vi "DBM Reg proc_temp.vi"(4 "Calfunc ?":bool, 6 "배열":u32[](array[numeric]), 7 "Query info":T1, 8 "에러 입력":errorcluster caption="에러 입력(에러 없음)", 9 "CMC":string[][](array[string]), 10 "calfunc":string[][](array[string]), 11 "Proc 참조 in":refnum<vi>) -> (0 "에러 출력":errorcluster, 2 "배열출력":string[][](array[string]), 3 "에러?":bool)   [LabVIEW 2020]
uses:
  Controls/Clst_Query Info.ctl
  Public/Polymorph/Array Dedup_2D Str.vi
  Public/Polymorph/Array Dedup_1D Str.vi
  <vilib>/Utility/error.llb/Error Cluster From Error Code.vi
  Public/Polymorph/Cell Space_Table.vi
  <vilib>/ErrorRing/Error Ring.xnode
panel:
  out "값":string[][](array[string])
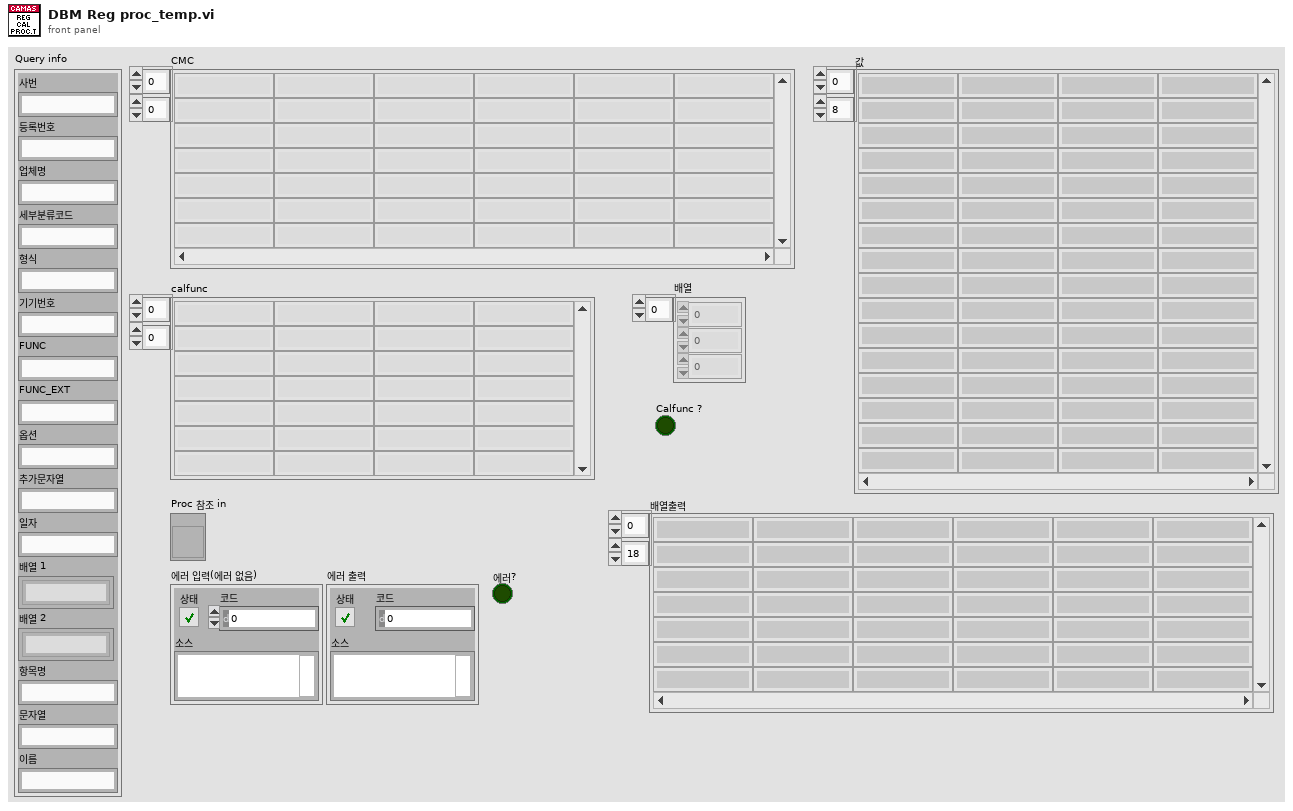
[diagram p1: front panel]
types:
  T1 = typedef "Clst_Query Info.ctl" = cluster{"사번":string, "등록번호":string, "업체명":string, "세부분류코드":string, "형식":string, "기기번호":string, "FUNC":string, "FUNC_EXT":string, "옵션":string, "추가문자열":string, "일자":string, "배열 1":string[], "배열 2":string[], "항목명":string, "문자열":string, "이름":string}
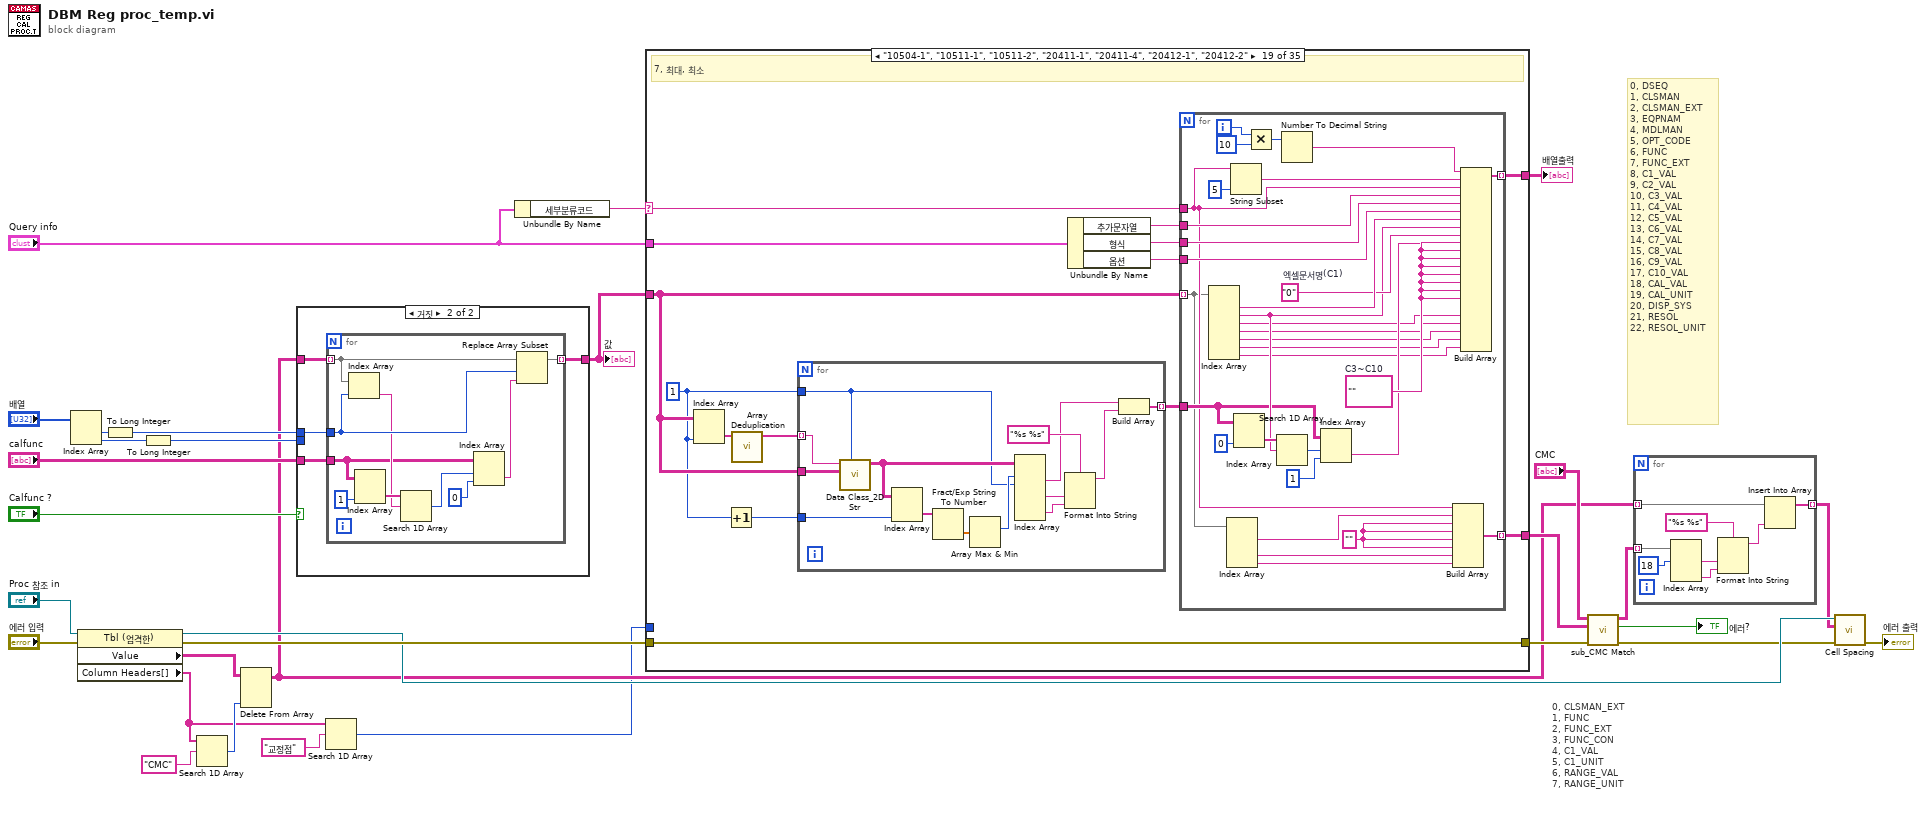
[diagram p0: block diagram]
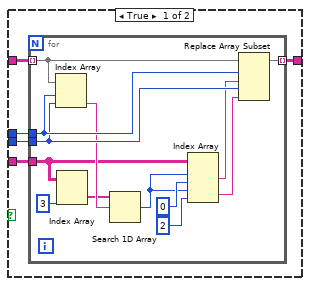
[diagram p2: hidden frame]
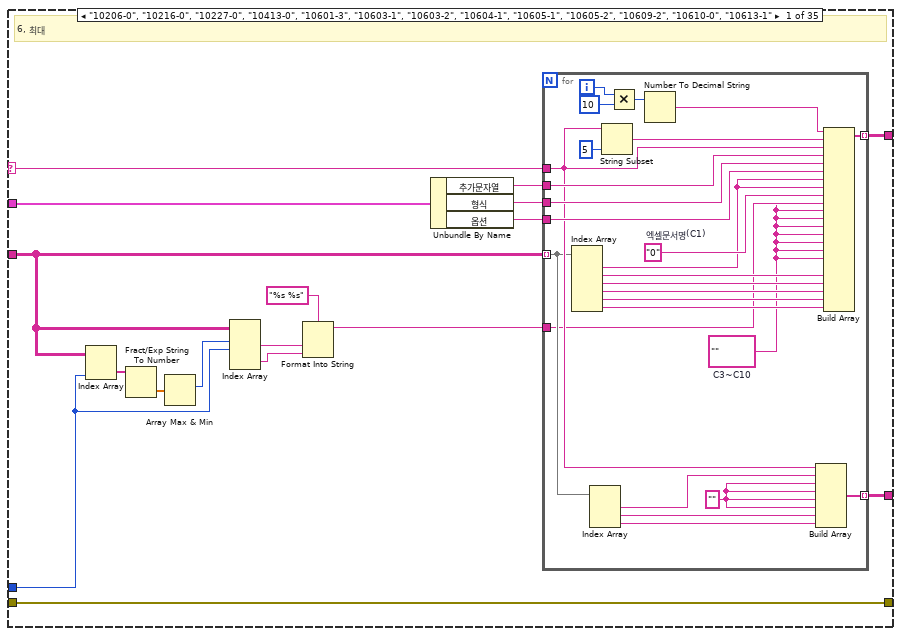
[diagram p3: hidden frame]
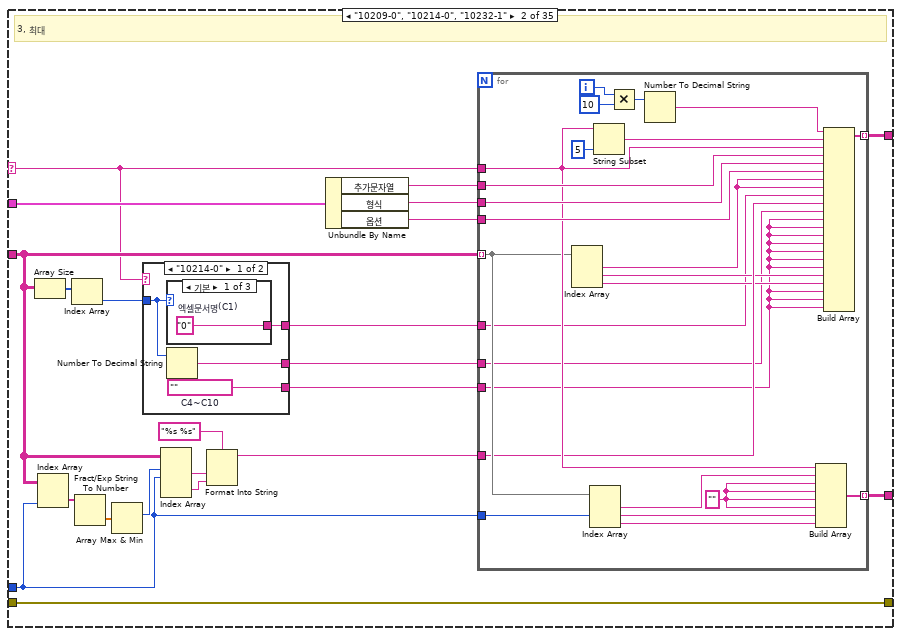
[diagram p4: hidden frame]
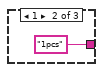
[diagram p5: hidden frame]
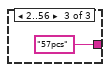
[diagram p6: hidden frame]
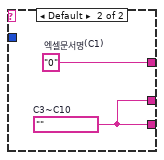
[diagram p7: hidden frame]
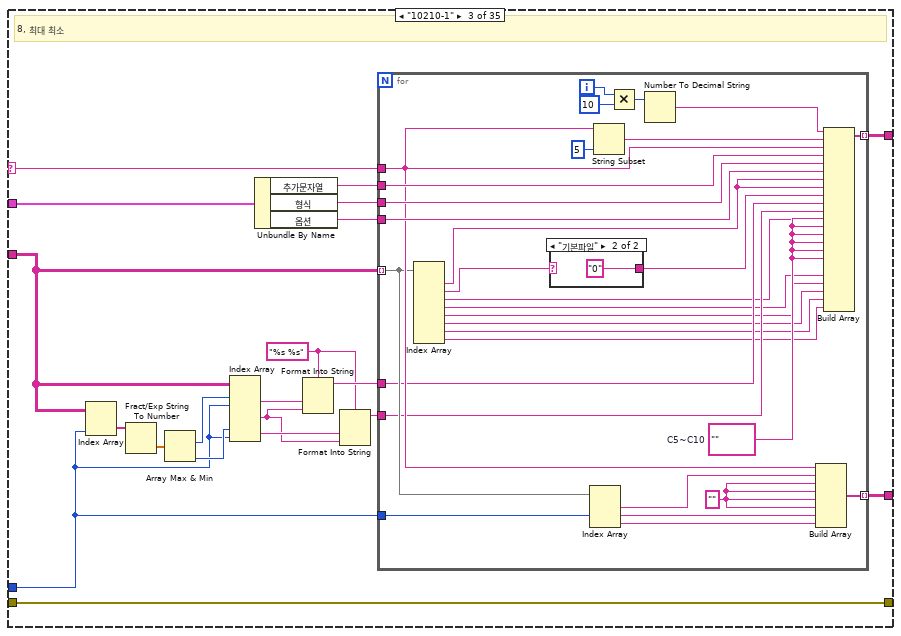
[diagram p8: hidden frame]
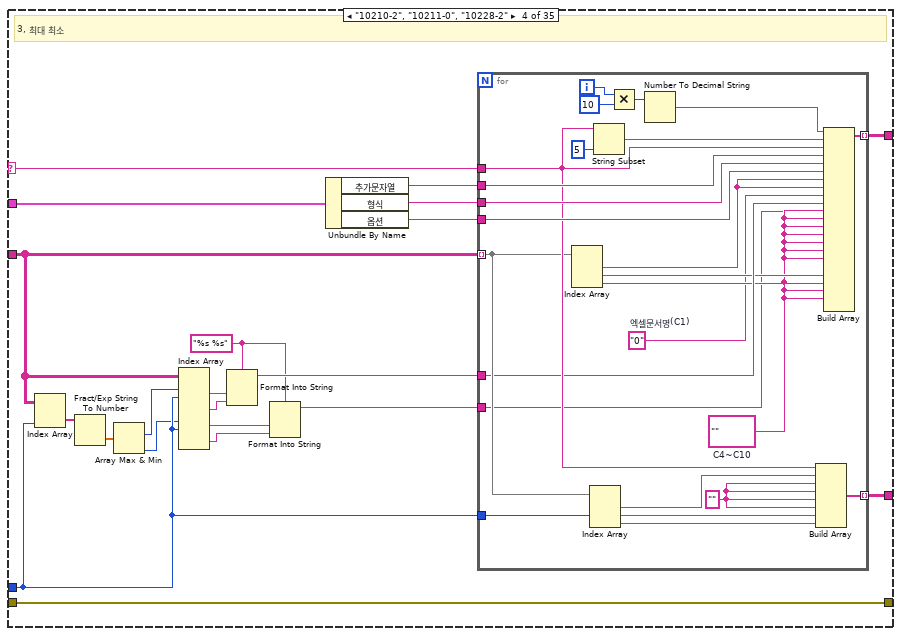
[diagram p10: hidden frame]
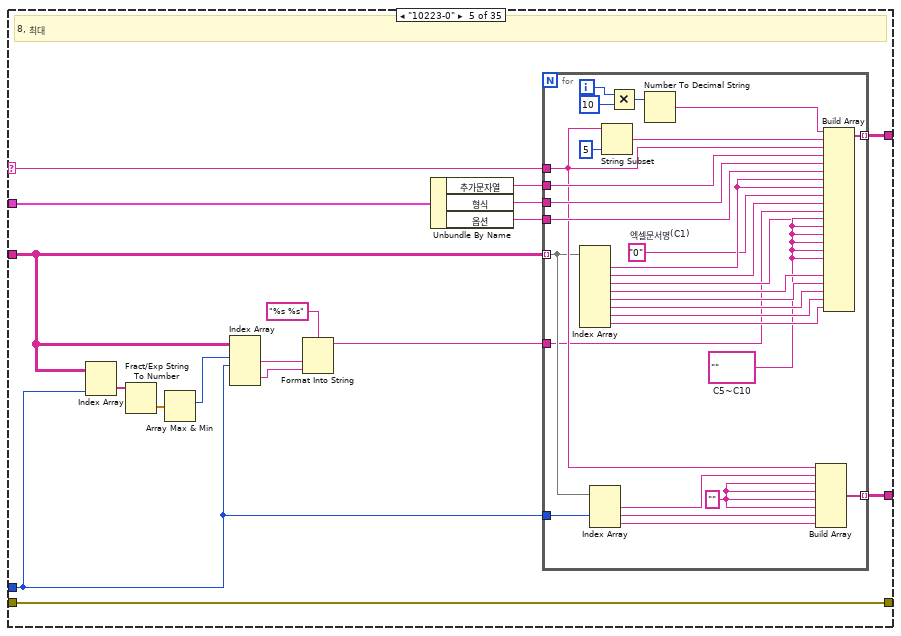
[diagram p11: hidden frame]
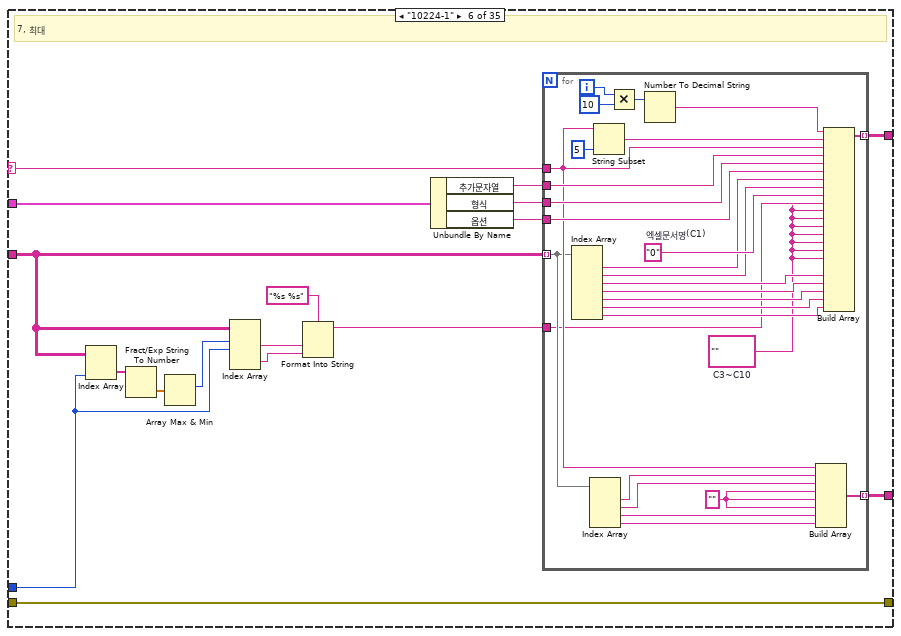
[diagram p12: hidden frame]
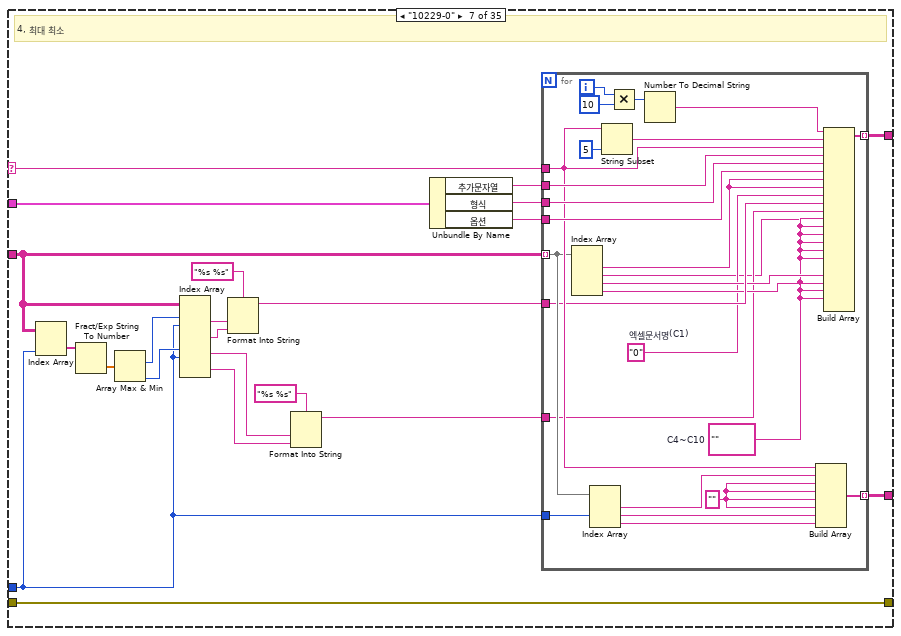
[diagram p13: hidden frame]
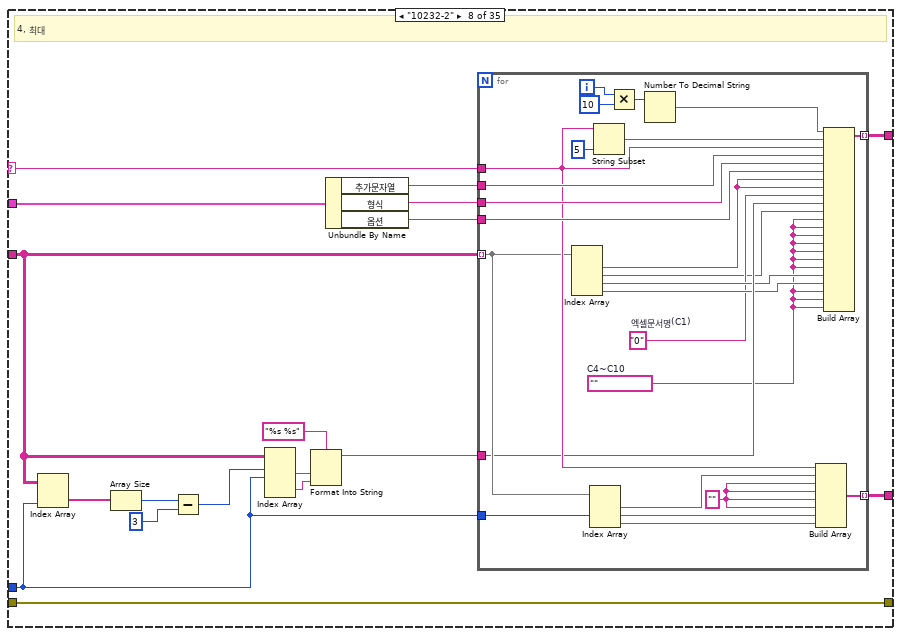
[diagram p14: hidden frame]
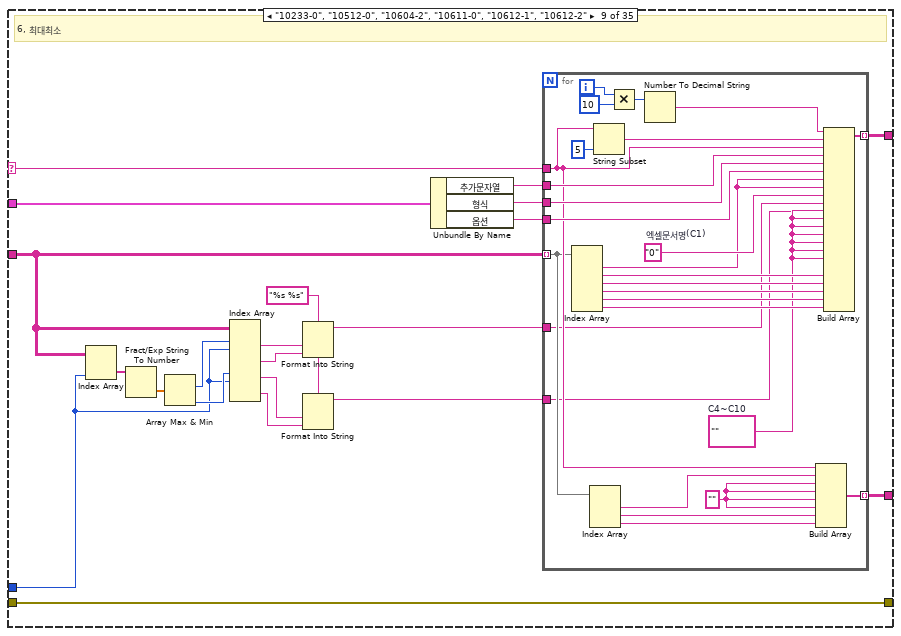
[diagram p15: hidden frame]
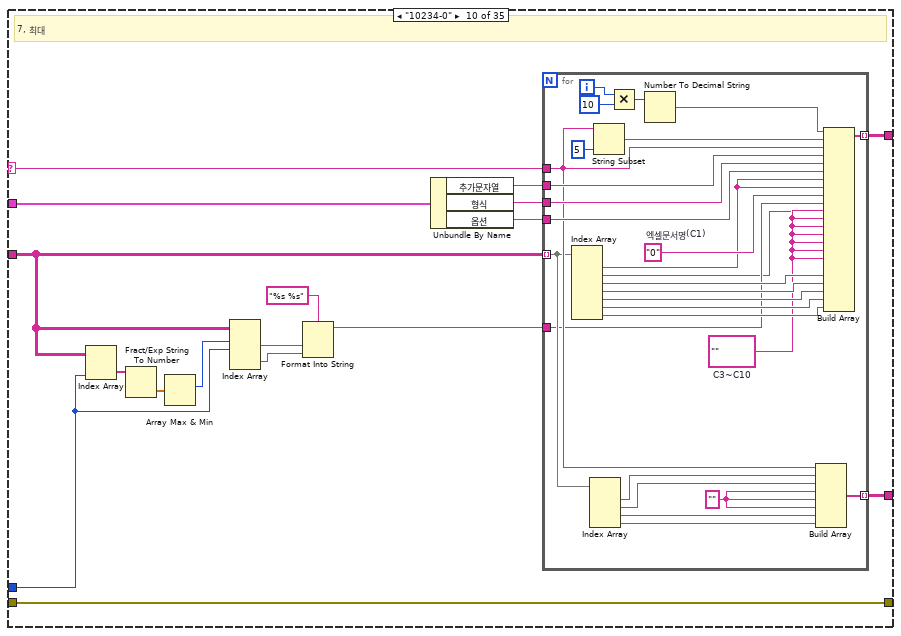
[diagram p16: hidden frame]
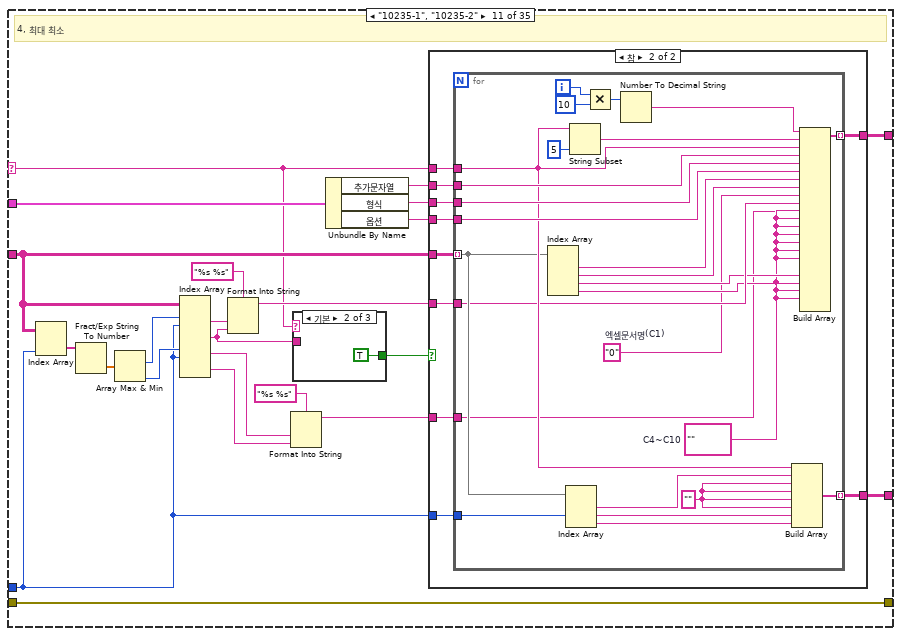
[diagram p17: hidden frame]
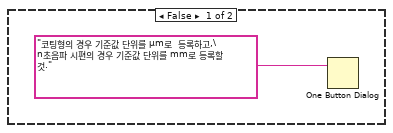
[diagram p18: hidden frame]
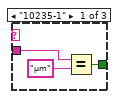
[diagram p19: hidden frame]
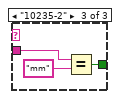
[diagram p20: hidden frame]
diagram:
  # "0, CLSMAN_EXT\n1, FUNC\n2, FUNC_EXT\n3, FUNC_CON\n4, C1_VAL\n5, C1_UNIT\n6, RANGE_VAL\n7, RANGE_UNIT"
  # "0, DSEQ\n1, CLSMAN\n2, CLSMAN_EXT\n3, EQPNAM\n4, MDLMAN\n5, OPT_CODE\n6, FUNC\n7, FUNC_EXT\n8, C1_VAL\n9, C2_VAL\n10, C3_VAL\n11, C4_VAL\n12, C5_VAL\n13, C6_VAL\n14, C7_VAL\n15, C8_VAL\n16, C9_VAL\n17, C10_VAL\n18, CAL_VAL\n19, CAL_UNIT\n20, DISP_SYS\n21, RESOL\n22, RESOL_UNIT"
  n1 = Index Array(array="배열") -> (element #1=w12:u32, element #2=w11:u32)  [unwired: 2 in]
  n2 = property class="Tbl (엄격한)"(reference="Proc 참조 in", error in="에러 입력") -> (reference out=w24:refnum<vi>, error out=w27:errorcluster, "Value"=w4:string[][], "Column Headers[]"=w2:string[])
  n3 = To Long Integer(number=w12) -> (32bit integer=w9:i32)
  n4 = To Long Integer(number=w11) -> (32bit integer=w8:i32)
  n5 = Search 1D Array(1D array=w2, element="CMC" ("원소")) -> (index of element=w22:i32)  [unwired: 1 in]
  n6 = Delete From Array(array=w4, index (col)=w22) -> (array with subset deleted=w5:string[][])  [unwired: 2 in, 1 out]
  n7 = case shown="거짓" "Calfunc ?" {
    tunnel: "calfunc" -> [w35 w52]
    tunnel: w5 -> [w34 w51]
    tunnel: w9 -> [w33 w50]
    tunnel: w8 -> [w32 _]
    tunnel: [w31 w49] -> w6
    frame True {
      n8 = for {
        tunnel: w34 -> [w43] mode=indexing
        tunnel: w35 -> [w42]
        tunnel: [w48] -> w31 mode=indexing
        tunnel: w33 -> [w47]
        tunnel: w32 -> [w46]
        n9 = Index Array(array=w43, index #1=w47, index #2=w46) -> (element #2=w45:string)  [unwired: 1 out]
        n10 = Index Array(array=w42, index (col)=3 ("인덱스 (열)")) -> (element=w44:string[])  [unwired: 1 in]
        n11 = Search 1D Array(1D array=w44, element=w45) -> (index of element=w36:i32)  [unwired: 1 in]
        n12 = Index Array(array=w42, index (row) #1=w36, index (col) #1=0 ("비활성화된 인덱스 (열)"), index (row) #2=w36, index (col) #2=2 ("비활성화된 인덱스 (열)")) -> (element #1=w40:string, element #2=w39:string)
        n13 = Replace Array Subset(array=w43, new element #1=w40, index #1=w47, new element #2=w39, index #2=w46) -> (w48:string[])
      }
    }
    frame False {
      n14 = for {
        tunnel: w51 -> [w58] mode=indexing
        tunnel: w52 -> [w57]
        tunnel: [w62] -> w49 mode=indexing
        tunnel: w50 -> [w61]
        n15 = Index Array(array=w58, index=w61) -> (element=w59:string)
        n16 = Index Array(array=w57, index (col)=1 ("비활성화된 인덱스 (열)")) -> (element=w60:string[])  [unwired: 1 in]
        n17 = Search 1D Array(1D array=w60, element=w59) -> (index of element=w56:i32)  [unwired: 1 in]
        n18 = Index Array(array=w57, index (row)=w56, index (col)=0 ("비활성화된 인덱스 (열)")) -> (element=w54:string)
        n19 = Replace Array Subset(array=w58, new element=w54, index=w61) -> (w62:string[])
      }
    }
  }
  "값" <- w6
  n20 = Search 1D Array(1D array=w2, element="교정점" ("원소")) -> (index of element=w1:i32)  [unwired: 1 in]
  n21 = Unbundle By Name("Query info") -> ("세부분류코드"=w28:string)
  n22 = case shown="\"10504-1\", \"10511-1\", \"10511-2\", \"20411-1\", \"20411-4\", \"20412-1\", \"20412-2\"" w28 {
    selector: w28 -> [w74 w109 w176 w229 w271 w317 w356 w403 w457 w501 w541 w613 w659 w706 w760 w849 w886 w927 w991 w1055 w1119 w1157 w1216 w1250 w1308 w1413 w1481 w1546 w1611 w1683 w1755 w1822 w1882 w1942 w1979]
    tunnel: [w72 w121 w174 w227 w269 w315 w366 w410 w455 w499 w551 w611 w657 w704 w758 w847 w884 w926 w989 w1053 w1117 w1155 w1214 w1248 w1306 w1411 w1479 w1544 w1609 w1681 w1753 w1820 w1880 w1940 w1981] -> w20
    tunnel: w27 -> [w72 w121 w174 w227 w269 w315 w366 w410 w455 w499 w551 w611 w657 w704 w758 w847 w884 w926 w989 w1053 w1117 w1155 w1214 w1248 w1306 w1411 w1479 w1544 w1609 w1681 w1753 w1820 w1880 w1940 _]
    tunnel: "Query info" -> [w79 w127 w181 w234 w276 w322 w372 w416 w462 w506 w557 w618 w664 w711 w765 w854 w891 w929 w1000 w1060 w1124 w1166 w1222 w1256 w1316 w1422 w1490 w1555 w1620 w1692 w1764 w1831 w1891 w1948 _]
    tunnel: w6 -> [w69 w112 w171 w225 w265 w311 w358 w404 w452 w495 w543 w607 w653 w700 w743 w846 w883 w923 w995 w1050 w1109 w1161 w1218 w1252 w1297 w1417 w1485 w1550 w1615 w1687 w1759 w1826 w1886 w1944 _]
    tunnel: [w75 w123 w177 w230 w272 w318 w368 w412 w458 w502 w553 w614 w660 w707 w761 w850 w887 w928 w992 w1056 w1120 w1158 w1217 w1251 w1309 w1414 w1482 w1547 w1612 w1684 w1756 w1823 w1883 w1943 _] -> w30
    tunnel: [w73 w122 w175 w228 w270 w316 w367 w411 w456 w500 w552 w612 w658 w705 w759 w848 w885 w915 w990 w1054 w1118 w1156 w1215 w1249 w1307 w1412 w1480 w1545 w1610 w1682 w1754 w1821 w1881 w1941 string[][] [] ("Value")] -> w16
    tunnel: w1 -> [w63 w114 w162 w219 w260 w306 w353 w405 w442 w490 w537 w602 w648 w695 w751 _ _ w925 _ w1051 w1108 _ _ _ _ _ _ _ _ _ _ _ _ _ _]
    frame "10206-0", "10216-0", "10227-0", "10413-0", "10601-3", "10603-1", "10603-2", "10604-1", "10605-1", "10605-2", "10609-2", "10610-0", "10613-1" {
      # "6, 최대"
      n23 = Index Array(array=w69, index (col)=w63) -> (element=w70:string[])  [unwired: 1 in]
      n24 = Fract/Exp String To Number(string=w70) -> (number=w71:dbl[])  [unwired: 3 in, 1 out]
      n25 = Array Max & Min(array=w71) -> (max index (indices)=w68:i32)  [unwired: 3 out]
      n26 = Index Array(array=w69, index (row) #1=w68, index (col) #1=w63) -> (element #1=w67:string, element #2=w64:string)  [unwired: 2 in]
      n27 = Format Into String(format string="%s %s" ("포맷 문자열"), w67, w64) -> (resulting string=w66:string)  [unwired: 2 in, 1 out]
      n28 = Unbundle By Name(w79) -> ("추가문자열"=w78:string, "형식"=w77:string, "옵션"=w76:string)
      n29 = for {
        tunnel: w69 -> [w88] mode=indexing
        tunnel: w74 -> [w89]
        tunnel: w78 -> [w98]
        tunnel: w77 -> [w97]
        tunnel: w76 -> [w96]
        tunnel: [w87] -> w73 mode=indexing
        tunnel: w66 -> [w84]
        tunnel: [w99] -> w75 mode=indexing
        i -> [w105]
        w85 = "" ("원소")
        w80 = ""  # C3~C10
        w95 = "0"  # 엑셀문서명(C1)
        n30 = Index Array(array=w88) -> (element #1=w83:string, element #2=w94:string, element #3=w93:string, element #4=w92:string, element #5=w91:string, element #6=w90:string)  [unwired: 6 in]
        n31 = Index Array(array=w88) -> (element #1=w86:string, element #2=w82:string, element #3=w81:string)  [unwired: 3 in]
        n32 = String Subset(string=w89, length (rest)=5 ("길이(나머지)")) -> (substring=w100:string)  [unwired: 1 in]
        n33 = Multiply(x=w105, y=10) -> (x*y=w103:i32)
        n34 = Number To Decimal String(number=w103) -> (decimal integer string=w102:string)  [unwired: 1 in]
        n35 = Build Array(w89, w86, w85, w85, w85, w85, w82, w81) -> (w87:string[])
        n36 = Build Array(w102, w100, w89, w98, w97, w96, w83, w83, w95, w84, w80, w80, w80, w80, w80, w80, w80, w80, w94, w93, w92, w91, w90) -> (w99:string[])
      }
    }
    frame "10209-0", "10214-0", "10232-1" {
      # "3, 최대"
      n37 = Array Size(array=w112) -> (size(s)=w111:i32[])
      n38 = Index Array(array=w112, index (col)=w114) -> (element=w113:string[])  [unwired: 1 in]
      n39 = Index Array(array=w111) -> (element=w110:i32)  [unwired: 1 in]
      n40 = Fract/Exp String To Number(string=w113) -> (number=w120:dbl[])  [unwired: 3 in, 1 out]
      n41 = Array Max & Min(array=w120) -> (max index (indices)=w118:i32)  [unwired: 3 out]
      n42 = case shown="\"10214-0\"" w109 {
        tunnel: [w131 w135] -> w108
        tunnel: [w130 w135] -> w106
        tunnel: w110 -> [w129 _]
        tunnel: [w128 w136] -> w107
        frame "10214-0" {
          w130 = ""  # C4~C10
          n43 = case shown="기본" w129 {
            tunnel: [w132 "1pcs" ("엑셀문서명(C1)") "57pcs" ("엑셀문서명(C1)")] -> w128
            frame Default {
              w132 = "0"  # 엑셀문서명(C1)
            }
            frame 1 {
            }
            frame 2..56 {
            }
          }
          n44 = Number To Decimal String(number=w129) -> (decimal integer string=w131:string)  [unwired: 1 in]
        }
        frame Default {
          w136 = "0"  # 엑셀문서명(C1)
          w135 = ""  # C3~C10
        }
      }
      n45 = Index Array(array=w112, index (row) #1=w118, index (col) #1=w114) -> (element #1=w117:string, element #2=w116:string)  [unwired: 2 in]
      n46 = Format Into String(format string="%s %s" ("포맷 문자열"), w117, w116) -> (resulting string=w115:string)  [unwired: 2 in, 1 out]
      n47 = Unbundle By Name(w127) -> ("추가문자열"=w126:string, "형식"=w125:string, "옵션"=w124:string)
      n48 = for {
        tunnel: w112 -> [w150] mode=indexing
        tunnel: w109 -> [w151]
        tunnel: w126 -> [w154]
        tunnel: w125 -> [w153]
        tunnel: w124 -> [w152]
        tunnel: [w149] -> w122 mode=indexing
        tunnel: w115 -> [w147]
        tunnel: [w155] -> w123 mode=indexing
        tunnel: w114 -> [w144]
        tunnel: w108 -> [w139]
        tunnel: w107 -> [w138]
        tunnel: w106 -> [w137]
        i -> [w161]
        w143 = "" ("원소")
        n49 = Index Array(array=w150) -> (element #1=w142:string, element #2=w141:string, element #3=w140:string)  [unwired: 3 in]
        n50 = Index Array(array=w150, index #2=w144) -> (element #1=w148:string, element #2=w146:string, element #3=w145:string)  [unwired: 2 in]
        n51 = String Subset(string=w151, length (rest)=5 ("길이(나머지)")) -> (substring=w156:string)  [unwired: 1 in]
        n52 = Multiply(x=w161, y=10) -> (x*y=w159:i32)
        n53 = Number To Decimal String(number=w159) -> (decimal integer string=w158:string)  [unwired: 1 in]
        n54 = Build Array(w151, w148, w143, w143, w143, w143, w146, w145) -> (w149:string[])
        n55 = Build Array(w158, w156, w151, w154, w153, w152, w142, w142, w138, w147, w139, w137, w137, w137, w137, w137, w137, w137, w141, w140, w137, w137, w137) -> (w155:string[])
      }
    }
    frame "10210-1" {
      w166 = "%s %s" ("포맷 문자열")
      # "8, 최대 최소"
      n56 = Index Array(array=w171, index (col)=w162) -> (element=w172:string[])  [unwired: 1 in]
      n57 = Fract/Exp String To Number(string=w172) -> (number=w173:dbl[])  [unwired: 3 in, 1 out]
      n58 = Array Max & Min(array=w173) -> (max index (indices)=w170:i32, min index (indices)=w167:i32)  [unwired: 2 out]
      n59 = Index Array(array=w171, index (row) #1=w170, index (col) #1=w162, index (row) #3=w167, index (col) #3=w162) -> (element #1=w169:string, element #2=w164:string, element #3=w165:string)  [unwired: 2 in]
      n60 = Unbundle By Name(w181) -> ("추가문자열"=w180:string, "형식"=w179:string, "옵션"=w178:string)
      n61 = Format Into String(format string=w166, w169, w164) -> (resulting string=w168:string)  [unwired: 2 in, 1 out]
      n62 = Format Into String(format string=w166, w165, w164) -> (resulting string=w163:string)  [unwired: 2 in, 1 out]
      n63 = for {
        tunnel: w171 -> [w200] mode=indexing
        tunnel: w176 -> [w201]
        tunnel: w180 -> [w204]
        tunnel: w179 -> [w203]
        tunnel: w178 -> [w202]
        tunnel: [w199] -> w175 mode=indexing
        tunnel: w168 -> [w196]
        tunnel: [w205] -> w177 mode=indexing
        tunnel: w163 -> [w192]
        tunnel: w162 -> [w185]
        i -> [w211]
        w197 = "" ("원소")
        w195 = ""  # C5~C10
        n64 = Index Array(array=w200) -> (element #1=w184:string, element #2=w183:string, element #3=w191:string, element #4=w190:string, element #5=w189:string, element #6=w188:string, element #7=w187:string, element #8=w186:string)  [unwired: 8 in]
        n65 = case shown="\"기본파일\"" w183 {
          selector: w183 -> [w212 _]
          tunnel: [w212 "0" ("원소")] -> w182
          frame Default {
          }
          frame "기본파일" {
          }
        }
        n66 = Index Array(array=w200, index #2=w185) -> (element #1=w198:string, element #2=w194:string, element #3=w193:string)  [unwired: 2 in]
        n67 = String Subset(string=w201, length (rest)=5 ("길이(나머지)")) -> (substring=w206:string)  [unwired: 1 in]
        n68 = Multiply(x=w211, y=10) -> (x*y=w209:i32)
        n69 = Number To Decimal String(number=w209) -> (decimal integer string=w208:string)  [unwired: 1 in]
        n70 = Build Array(w201, w198, w197, w197, w197, w197, w194, w193) -> (w199:string[])
        n71 = Build Array(w208, w206, w201, w204, w203, w202, w184, w184, w182, w196, w192, w191, w195, w195, w195, w195, w195, w195, w190, w189, w188, w187, w186) -> (w205:string[])
      }
    }
    frame "10210-2", "10211-0", "10228-2" {
      w215 = "%s %s" ("포맷 문자열")
      # "3, 최대 최소"
      n72 = Index Array(array=w225, index (col)=w219) -> (element=w220:string[])  [unwired: 1 in]
      n73 = Fract/Exp String To Number(string=w220) -> (number=w226:dbl[])  [unwired: 3 in, 1 out]
      n74 = Array Max & Min(array=w226) -> (max index (indices)=w224:i32, min index (indices)=w218:i32)  [unwired: 2 out]
      n75 = Index Array(array=w225, index (row) #1=w224, index (col) #1=w219, index (row) #3=w218, index (col) #3=w219) -> (element #1=w223:string, element #2=w222:string, element #3=w217:string, element #4=w216:string)  [unwired: 4 in]
      n76 = Format Into String(format string=w215, w223, w222) -> (resulting string=w221:string)  [unwired: 2 in, 1 out]
      n77 = Format Into String(format string=w215, w217, w216) -> (resulting string=w214:string)  [unwired: 2 in, 1 out]
      n78 = Unbundle By Name(w234) -> ("추가문자열"=w233:string, "형식"=w232:string, "옵션"=w231:string)
      n79 = for {
        tunnel: w225 -> [w248] mode=indexing
        tunnel: w229 -> [w249]
        tunnel: w233 -> [w252]
        tunnel: w232 -> [w251]
        tunnel: w231 -> [w250]
        tunnel: [w247] -> w228 mode=indexing
        tunnel: w221 -> [w245]
        tunnel: [w253] -> w230 mode=indexing
        tunnel: w219 -> [w242]
        tunnel: w214 -> [w235]
        i -> [w259]
        w236 = "0"  # 엑셀문서명(C1)
        w241 = "" ("원소")
        w237 = ""  # C4~C10
        n80 = Index Array(array=w248) -> (element #1=w240:string, element #2=w239:string, element #3=w238:string)  [unwired: 3 in]
        n81 = Index Array(array=w248, index #2=w242) -> (element #1=w246:string, element #2=w244:string, element #3=w243:string)  [unwired: 2 in]
        n82 = String Subset(string=w249, length (rest)=5 ("길이(나머지)")) -> (substring=w254:string)  [unwired: 1 in]
        n83 = Multiply(x=w259, y=10) -> (x*y=w257:i32)
        n84 = Number To Decimal String(number=w257) -> (decimal integer string=w256:string)  [unwired: 1 in]
        n85 = Build Array(w249, w246, w241, w241, w241, w241, w244, w243) -> (w247:string[])
        n86 = Build Array(w256, w254, w249, w252, w251, w250, w240, w240, w236, w245, w235, w237, w237, w237, w237, w237, w237, w237, w239, w238, w237, w237, w237) -> (w253:string[])
      }
    }
    frame "10223-0" {
      # "8, 최대"
      n87 = Index Array(array=w265, index (col)=w260) -> (element=w267:string[])  [unwired: 1 in]
      n88 = Fract/Exp String To Number(string=w267) -> (number=w268:dbl[])  [unwired: 3 in, 1 out]
      n89 = Array Max & Min(array=w268) -> (max index (indices)=w264:i32)  [unwired: 3 out]
      n90 = Index Array(array=w265, index (row) #1=w264, index (col) #1=w260) -> (element #1=w263:string, element #2=w262:string)  [unwired: 2 in]
      n91 = Format Into String(format string="%s %s" ("포맷 문자열"), w263, w262) -> (resulting string=w261:string)  [unwired: 2 in, 1 out]
      n92 = Unbundle By Name(w276) -> ("추가문자열"=w275:string, "형식"=w274:string, "옵션"=w273:string)
      n93 = for {
        tunnel: w265 -> [w294] mode=indexing
        tunnel: w271 -> [w295]
        tunnel: w275 -> [w298]
        tunnel: w274 -> [w297]
        tunnel: w273 -> [w296]
        tunnel: [w293] -> w270 mode=indexing
        tunnel: w261 -> [w279]
        tunnel: [w299] -> w272 mode=indexing
        tunnel: w260 -> [w284]
        i -> [w305]
        w282 = "" ("원소")
        w283 = ""  # C5~C10
        w278 = "0"  # 엑셀문서명(C1)
        n94 = Index Array(array=w294) -> (element #1=w281:string, element #2=w277:string, element #3=w280:string, element #4=w291:string, element #5=w290:string, element #6=w289:string, element #7=w288:string, element #8=w287:string)  [unwired: 8 in]
        n95 = Index Array(array=w294, index #2=w284) -> (element #1=w292:string, element #2=w286:string, element #3=w285:string)  [unwired: 2 in]
        n96 = String Subset(string=w295, length (rest)=5 ("길이(나머지)")) -> (substring=w300:string)  [unwired: 1 in]
        n97 = Multiply(x=w305, y=10) -> (x*y=w303:i32)
        n98 = Number To Decimal String(number=w303) -> (decimal integer string=w302:string)  [unwired: 1 in]
        n99 = Build Array(w295, w292, w282, w282, w282, w282, w286, w285) -> (w293:string[])
        n100 = Build Array(w302, w300, w295, w298, w297, w296, w281, w281, w278, w277, w279, w280, w283, w283, w283, w283, w283, w283, w291, w290, w289, w288, w287) -> (w299:string[])
      }
    }
    frame "10224-1" {
      # "7, 최대"
      n101 = Index Array(array=w311, index (col)=w306) -> (element=w313:string[])  [unwired: 1 in]
      n102 = Fract/Exp String To Number(string=w313) -> (number=w314:dbl[])  [unwired: 3 in, 1 out]
      n103 = Array Max & Min(array=w314) -> (max index (indices)=w310:i32)  [unwired: 3 out]
      n104 = Index Array(array=w311, index (row) #1=w310, index (col) #1=w306) -> (element #1=w309:string, element #2=w308:string)  [unwired: 2 in]
      n105 = Format Into String(format string="%s %s" ("포맷 문자열"), w309, w308) -> (resulting string=w307:string)  [unwired: 2 in, 1 out]
      n106 = Unbundle By Name(w322) -> ("추가문자열"=w321:string, "형식"=w320:string, "옵션"=w319:string)
      n107 = for {
        tunnel: w311 -> [w333] mode=indexing
        tunnel: w317 -> [w334]
        tunnel: w321 -> [w343]
        tunnel: w320 -> [w342]
        tunnel: w319 -> [w341]
        tunnel: [w332] -> w316 mode=indexing
        tunnel: w307 -> [w328]
        tunnel: [w344] -> w318 mode=indexing
        i -> [w350]
        w329 = "" ("원소")
        w326 = ""  # C3~C10
        w340 = "0"  # 엑셀문서명(C1)
        n108 = Index Array(array=w333) -> (element #1=w327:string, element #2=w325:string, element #3=w339:string, element #4=w338:string, element #5=w337:string, element #6=w336:string, element #7=w335:string)  [unwired: 7 in]
        n109 = Index Array(array=w333) -> (element #1=w324:string, element #2=w323:string, element #3=w331:string, element #4=w330:string)  [unwired: 4 in]
        n110 = String Subset(string=w334, length (rest)=5 ("길이(나머지)")) -> (substring=w345:string)  [unwired: 1 in]
        n111 = Multiply(x=w350, y=10) -> (x*y=w348:i32)
        n112 = Number To Decimal String(number=w348) -> (decimal integer string=w347:string)  [unwired: 1 in]
        n113 = Build Array(w334, w324, w323, w329, w329, w329, w331, w330) -> (w332:string[])
        n114 = Build Array(w347, w345, w334, w343, w342, w341, w327, w325, w340, w328, w326, w326, w326, w326, w326, w326, w326, w326, w339, w338, w337, w336, w335) -> (w344:string[])
      }
    }
    frame "10229-0" {
      # "4, 최대 최소"
      n115 = Index Array(array=w358, index (col)=w353) -> (element=w360:string[])  [unwired: 1 in]
      n116 = Fract/Exp String To Number(string=w360) -> (number=w365:dbl[])  [unwired: 3 in, 1 out]
      n117 = Array Max & Min(array=w365) -> (max index (indices)=w363:i32, min index (indices)=w354:i32)  [unwired: 2 out]
      n118 = Index Array(array=w358, index (row) #1=w363, index (col) #1=w353, index (row) #3=w354, index (col) #3=w353) -> (element #1=w362:string, element #2=w355:string, element #3=w352:string, element #4=w351:string)  [unwired: 4 in]
      n119 = Format Into String(format string="%s %s" ("포맷 문자열"), w362, w355) -> (resulting string=w361:string)  [unwired: 2 in, 1 out]
      n120 = Format Into String(format string="%s %s" ("포맷 문자열"), w352, w351) -> (resulting string=w357:string)  [unwired: 2 in, 1 out]
      n121 = Unbundle By Name(w372) -> ("추가문자열"=w371:string, "형식"=w370:string, "옵션"=w369:string)
      n122 = for {
        tunnel: w358 -> [w387] mode=indexing
        tunnel: w356 -> [w388]
        tunnel: w371 -> [w391]
        tunnel: w370 -> [w390]
        tunnel: w369 -> [w389]
        tunnel: [w386] -> w367 mode=indexing
        tunnel: w361 -> [w384]
        tunnel: [w392] -> w368 mode=indexing
        tunnel: w353 -> [w375]
        tunnel: w357 -> [w376]
        i -> [w398]
        w378 = "0"  # 엑셀문서명(C1)
        w381 = "" ("원소")
        w377 = ""  # C4~C10
        n123 = Index Array(array=w387) -> (element #1=w374:string, element #2=w373:string, element #3=w380:string, element #4=w379:string)  [unwired: 4 in]
        n124 = Index Array(array=w387, index #2=w375) -> (element #1=w385:string, element #2=w383:string, element #3=w382:string)  [unwired: 2 in]
        n125 = String Subset(string=w388, length (rest)=5 ("길이(나머지)")) -> (substring=w393:string)  [unwired: 1 in]
        n126 = Multiply(x=w398, y=10) -> (x*y=w396:i32)
        n127 = Number To Decimal String(number=w396) -> (decimal integer string=w395:string)  [unwired: 1 in]
        n128 = Build Array(w388, w385, w381, w381, w381, w381, w383, w382) -> (w386:string[])
        n129 = Build Array(w395, w393, w388, w391, w390, w389, w374, w374, w378, w384, w376, w373, w377, w377, w377, w377, w377, w377, w380, w379, w377, w377, w377) -> (w392:string[])
      }
    }
    frame "10232-2" {
      # "4, 최대"
      n130 = Index Array(array=w404, index (col)=w405) -> (element=w402:string[])  [unwired: 1 in]
      n131 = Array Size(array=w402) -> (size(s)=w401:i32)
      n132 = Subtract(x=w401, y=3) -> (x-y=w399:i32)
      n133 = Index Array(array=w404, index (row) #1=w399, index (col) #1=w405) -> (element #1=w408:string, element #2=w407:string)  [unwired: 2 in]
      n134 = Format Into String(format string="%s %s" ("포맷 문자열"), w408, w407) -> (resulting string=w406:string)  [unwired: 2 in, 1 out]
      n135 = Unbundle By Name(w416) -> ("추가문자열"=w415:string, "형식"=w414:string, "옵션"=w413:string)
      n136 = for {
        tunnel: w404 -> [w430] mode=indexing
        tunnel: w403 -> [w431]
        tunnel: w415 -> [w434]
        tunnel: w414 -> [w433]
        tunnel: w413 -> [w432]
        tunnel: [w429] -> w411 mode=indexing
        tunnel: w406 -> [w427]
        tunnel: [w435] -> w412 mode=indexing
        tunnel: w405 -> [w424]
        i -> [w441]
        w419 = ""  # C4~C10
        w420 = "0"  # 엑셀문서명(C1)
        w423 = "" ("원소")
        n137 = Index Array(array=w430) -> (element #1=w418:string, element #2=w417:string, element #3=w422:string, element #4=w421:string)  [unwired: 4 in]
        n138 = Index Array(array=w430, index #2=w424) -> (element #1=w428:string, element #2=w426:string, element #3=w425:string)  [unwired: 2 in]
        n139 = String Subset(string=w431, length (rest)=5 ("길이(나머지)")) -> (substring=w436:string)  [unwired: 1 in]
        n140 = Multiply(x=w441, y=10) -> (x*y=w439:i32)
        n141 = Number To Decimal String(number=w439) -> (decimal integer string=w438:string)  [unwired: 1 in]
        n142 = Build Array(w431, w428, w423, w423, w423, w423, w426, w425) -> (w429:string[])
        n143 = Build Array(w438, w436, w431, w434, w433, w432, w418, w418, w420, w427, w417, w419, w419, w419, w419, w419, w419, w419, w422, w421, w419, w419, w419) -> (w435:string[])
      }
    }
    frame "10233-0", "10512-0", "10604-2", "10611-0", "10612-1", "10612-2" {
      w447 = "%s %s" ("포맷 문자열")
      # "6, 최대최소"
      n144 = Index Array(array=w452, index (col)=w442) -> (element=w453:string[])  [unwired: 1 in]
      n145 = Fract/Exp String To Number(string=w453) -> (number=w454:dbl[])  [unwired: 3 in, 1 out]
      n146 = Array Max & Min(array=w454) -> (max index (indices)=w451:i32, min index (indices)=w448:i32)  [unwired: 2 out]
      n147 = Index Array(array=w452, index (row) #1=w451, index (col) #1=w442, index (row) #3=w448, index (col) #3=w442) -> (element #1=w450:string, element #2=w445:string, element #3=w446:string, element #4=w443:string)  [unwired: 4 in]
      n148 = Format Into String(format string=w447, w450, w445) -> (resulting string=w449:string)  [unwired: 2 in, 1 out]
      n149 = Format Into String(format string=w447, w446, w443) -> (resulting string=w444:string)  [unwired: 2 in, 1 out]
      n150 = Unbundle By Name(w462) -> ("추가문자열"=w461:string, "형식"=w460:string, "옵션"=w459:string)
      n151 = for {
        tunnel: w452 -> [w472] mode=indexing
        tunnel: w457 -> [w473]
        tunnel: w461 -> [w482]
        tunnel: w460 -> [w481]
        tunnel: w459 -> [w480]
        tunnel: [w471] -> w456 mode=indexing
        tunnel: w449 -> [w468]
        tunnel: [w483] -> w458 mode=indexing
        tunnel: w444 -> [w463]
        i -> [w489]
        w469 = "" ("원소")
        w467 = ""  # C4~C10
        w479 = "0"  # 엑셀문서명(C1)
        n152 = Index Array(array=w472) -> (element #1=w466:string, element #2=w478:string, element #3=w477:string, element #4=w476:string, element #5=w475:string, element #6=w474:string)  [unwired: 6 in]
        n153 = Index Array(array=w472) -> (element #1=w470:string, element #2=w465:string, element #3=w464:string)  [unwired: 3 in]
        n154 = String Subset(string=w473, length (rest)=5 ("길이(나머지)")) -> (substring=w484:string)  [unwired: 1 in]
        n155 = Multiply(x=w489, y=10) -> (x*y=w487:i32)
        n156 = Number To Decimal String(number=w487) -> (decimal integer string=w486:string)  [unwired: 1 in]
        n157 = Build Array(w473, w470, w469, w469, w469, w469, w465, w464) -> (w471:string[])
        n158 = Build Array(w486, w484, w473, w482, w481, w480, w466, w466, w479, w468, w463, w467, w467, w467, w467, w467, w467, w467, w478, w477, w476, w475, w474) -> (w483:string[])
      }
    }
    frame "10234-0" {
      # "7, 최대"
      n159 = Index Array(array=w495, index (col)=w490) -> (element=w497:string[])  [unwired: 1 in]
      n160 = Fract/Exp String To Number(string=w497) -> (number=w498:dbl[])  [unwired: 3 in, 1 out]
      n161 = Array Max & Min(array=w498) -> (max index (indices)=w494:i32)  [unwired: 3 out]
      n162 = Index Array(array=w495, index (row) #1=w494, index (col) #1=w490) -> (element #1=w493:string, element #2=w492:string)  [unwired: 2 in]
      n163 = Format Into String(format string="%s %s" ("포맷 문자열"), w493, w492) -> (resulting string=w491:string)  [unwired: 2 in, 1 out]
      n164 = Unbundle By Name(w506) -> ("추가문자열"=w505:string, "형식"=w504:string, "옵션"=w503:string)
      n165 = for {
        tunnel: w495 -> [w517] mode=indexing
        tunnel: w501 -> [w518]
        tunnel: w505 -> [w527]
        tunnel: w504 -> [w526]
        tunnel: w503 -> [w525]
        tunnel: [w516] -> w500 mode=indexing
        tunnel: w491 -> [w512]
        tunnel: [w528] -> w502 mode=indexing
        i -> [w534]
        w513 = "" ("원소")
        w511 = ""  # C3~C10
        w524 = "0"  # 엑셀문서명(C1)
        n166 = Index Array(array=w517) -> (element #1=w508:string, element #2=w507:string, element #3=w523:string, element #4=w522:string, element #5=w521:string, element #6=w520:string, element #7=w519:string)  [unwired: 7 in]
        n167 = Index Array(array=w517) -> (element #1=w510:string, element #2=w509:string, element #3=w515:string, element #4=w514:string)  [unwired: 4 in]
        n168 = String Subset(string=w518, length (rest)=5 ("길이(나머지)")) -> (substring=w529:string)  [unwired: 1 in]
        n169 = Multiply(x=w534, y=10) -> (x*y=w532:i32)
        n170 = Number To Decimal String(number=w532) -> (decimal integer string=w531:string)  [unwired: 1 in]
        n171 = Build Array(w518, w510, w509, w513, w513, w513, w515, w514) -> (w516:string[])
        n172 = Build Array(w531, w529, w518, w527, w526, w525, w508, w508, w524, w512, w507, w511, w511, w511, w511, w511, w511, w511, w523, w522, w521, w520, w519) -> (w528:string[])
      }
    }
    frame "10235-1", "10235-2" {
      # "4, 최대 최소"
      n173 = Index Array(array=w543, index (col)=w537) -> (element=w545:string[])  [unwired: 1 in]
      n174 = Fract/Exp String To Number(string=w545) -> (number=w550:dbl[])  [unwired: 3 in, 1 out]
      n175 = Array Max & Min(array=w550) -> (max index (indices)=w548:i32, min index (indices)=w538:i32)  [unwired: 2 out]
      n176 = Index Array(array=w543, index (row) #1=w548, index (col) #1=w537, index (row) #3=w538, index (col) #3=w537) -> (element #1=w547:string, element #2=w540:string, element #3=w536:string, element #4=w535:string)  [unwired: 4 in]
      n177 = Format Into String(format string="%s %s" ("포맷 문자열"), w547, w540) -> (resulting string=w546:string)  [unwired: 2 in, 1 out]
      n178 = Format Into String(format string="%s %s" ("포맷 문자열"), w536, w535) -> (resulting string=w542:string)  [unwired: 2 in, 1 out]
      n179 = case shown="기본" w541 {
        tunnel: w540 -> [w596 _ w601]
        tunnel: [w595 TRUE w599] -> w539
        frame "10235-1" {
          n180 = Equal?(x=w596, y="μm") -> (x = y?=w595:bool)
        }
        frame Default {
        }
        frame "10235-2" {
          n181 = Equal?(x=w601, y="mm") -> (x = y?=w599:bool)
        }
      }
      n182 = Unbundle By Name(w557) -> ("추가문자열"=w556:string, "형식"=w555:string, "옵션"=w554:string)
      n183 = case shown="참" w539 {
        tunnel: w556 -> [_ w568]
        tunnel: w555 -> [_ w567]
        tunnel: w554 -> [_ w566]
        tunnel: [_ w565] -> w553
        tunnel: [_ w564] -> w552
        tunnel: w546 -> [_ w563]
        tunnel: w537 -> [_ w562]
        tunnel: w543 -> [_ w561]
        tunnel: w542 -> [_ w560]
        tunnel: w541 -> [_ w559]
        frame False {
          n184 = One Button Dialog(message="코팅형의 경우 기준값 단위를 μm로  등록하고,\n초음파 시편의 경우 기준값 단위를 mm로 등록할 것." ("메시지")) -> ()  [unwired: 1 in, 1 out]
        }
        frame True {
          n185 = for {
            tunnel: w561 -> [w583] mode=indexing
            tunnel: w559 -> [w584]
            tunnel: w568 -> [w587]
            tunnel: w567 -> [w586]
            tunnel: w566 -> [w585]
            tunnel: [w582] -> w564 mode=indexing
            tunnel: w563 -> [w580]
            tunnel: [w588] -> w565 mode=indexing
            tunnel: w562 -> [w570]
            tunnel: w560 -> [w571]
            i -> [w594]
            w573 = "0"  # 엑셀문서명(C1)
            w577 = "" ("원소")
            w572 = ""  # C4~C10
            n186 = Index Array(array=w583) -> (element #1=w569:string, element #2=w574:string, element #3=w576:string, element #4=w575:string)  [unwired: 4 in]
            n187 = Index Array(array=w583, index #2=w570) -> (element #1=w581:string, element #2=w579:string, element #3=w578:string)  [unwired: 2 in]
            n188 = String Subset(string=w584, length (rest)=5 ("길이(나머지)")) -> (substring=w589:string)  [unwired: 1 in]
            n189 = Multiply(x=w594, y=10) -> (x*y=w592:i32)
            n190 = Number To Decimal String(number=w592) -> (decimal integer string=w591:string)  [unwired: 1 in]
            n191 = Build Array(w584, w581, w577, w577, w577, w577, w579, w578) -> (w582:string[])
            n192 = Build Array(w591, w589, w584, w587, w586, w585, w569, w574, w573, w580, w571, w572, w572, w572, w572, w572, w572, w572, w576, w575, w572, w572, w572) -> (w588:string[])
          }
        }
      }
    }
    frame "10236-0", "10511-3" {
      # "8, 최대"
      n193 = Index Array(array=w607, index (col)=w602) -> (element=w609:string[])  [unwired: 1 in]
      n194 = Fract/Exp String To Number(string=w609) -> (number=w610:dbl[])  [unwired: 3 in, 1 out]
      n195 = Array Max & Min(array=w610) -> (max index (indices)=w606:i32)  [unwired: 3 out]
      n196 = Index Array(array=w607, index (row) #1=w606, index (col) #1=w602) -> (element #1=w605:string, element #2=w604:string)  [unwired: 2 in]
      n197 = Format Into String(format string="%s %s" ("포맷 문자열"), w605, w604) -> (resulting string=w603:string)  [unwired: 2 in, 1 out]
      n198 = Unbundle By Name(w618) -> ("추가문자열"=w617:string, "형식"=w616:string, "옵션"=w615:string)
      n199 = for {
        tunnel: w607 -> [w635] mode=indexing
        tunnel: w613 -> [w636]
        tunnel: w617 -> [w640]
        tunnel: w616 -> [w639]
        tunnel: w615 -> [w638]
        tunnel: [w634] -> w612 mode=indexing
        tunnel: w603 -> [w632]
        tunnel: [w641] -> w614 mode=indexing
        tunnel: w602 -> [w623]
        i -> [w647]
        w619 = "" ("원소")
        w620 = ""  # C4~C10
        w637 = "0"  # 엑셀문서명(C1)
        n200 = Index Array(array=w635) -> (element #1=w631:string, element #2=w622:string, element #3=w621:string, element #4=w630:string, element #5=w629:string, element #6=w628:string, element #7=w627:string, element #8=w626:string)  [unwired: 8 in]
        n201 = Index Array(array=w635, index #2=w623) -> (element #1=w633:string, element #2=w625:string, element #3=w624:string)  [unwired: 2 in]
        n202 = String Subset(string=w636, length (rest)=5 ("길이(나머지)")) -> (substring=w642:string)  [unwired: 1 in]
        n203 = Multiply(x=w647, y=10) -> (x*y=w645:i32)
        n204 = Number To Decimal String(number=w645) -> (decimal integer string=w644:string)  [unwired: 1 in]
        n205 = Build Array(w636, w633, w619, w619, w619, w619, w625, w624) -> (w634:string[])
        n206 = Build Array(w644, w642, w636, w640, w639, w638, w631, w622, w637, w632, w621, w620, w620, w620, w620, w620, w620, w620, w630, w629, w628, w627, w626) -> (w641:string[])
      }
    }
    frame "10304-2" {
      # "8, 최대"
      n207 = Index Array(array=w653, index (col)=w648) -> (element=w655:string[])  [unwired: 1 in]
      n208 = Fract/Exp String To Number(string=w655) -> (number=w656:dbl[])  [unwired: 3 in, 1 out]
      n209 = Array Max & Min(array=w656) -> (max index (indices)=w652:i32)  [unwired: 3 out]
      n210 = Index Array(array=w653, index (row) #1=w652, index (col) #1=w648) -> (element #1=w651:string, element #2=w650:string)  [unwired: 2 in]
      n211 = Format Into String(format string="%s %s" ("포맷 문자열"), w651, w650) -> (resulting string=w649:string)  [unwired: 2 in, 1 out]
      n212 = Unbundle By Name(w664) -> ("추가문자열"=w663:string, "형식"=w662:string, "옵션"=w661:string)
      n213 = for {
        tunnel: w653 -> [w682] mode=indexing
        tunnel: w659 -> [w683]
        tunnel: w663 -> [w687]
        tunnel: w662 -> [w686]
        tunnel: w661 -> [w685]
        tunnel: [w681] -> w658 mode=indexing
        tunnel: w649 -> [w678]
        tunnel: [w688] -> w660 mode=indexing
        tunnel: w648 -> [w666]
        i -> [w694]
        w679 = "" ("원소")
        w674 = ""  # C4~C10
        w684 = "0"  # 엑셀문서명(C1)
        n214 = Index Array(array=w682) -> (element #1=w677:string, element #2=w676:string, element #3=w675:string, element #4=w673:string, element #5=w672:string, element #6=w671:string, element #7=w670:string, element #8=w669:string)  [unwired: 8 in]
        n215 = Index Array(array=w682, index #2=w666) -> (element #1=w680:string, element #2=w668:string, element #3=w667:string)  [unwired: 2 in]
        n216 = String Subset(string=w683, length (rest)=5 ("길이(나머지)")) -> (substring=w689:string)  [unwired: 1 in]
        n217 = Multiply(x=w694, y=10) -> (x*y=w692:i32)
        n218 = Number To Decimal String(number=w692) -> (decimal integer string=w691:string)  [unwired: 1 in]
        n219 = Build Array(w683, w680, w679, "Angle" ("원소"), w679, w679, w668, w667) -> (w681:string[])
        n220 = Build Array(w691, w689, w683, w687, w686, w685, w677, w677, w684, w678, w676, w675, w674, w674, w674, w674, w674, w674, w673, w672, w671, w670, w669) -> (w688:string[])
      }
    }
    frame "10311-1" {
      # "9, 최대"
      n221 = Index Array(array=w700, index (col)=w695) -> (element=w702:string[])  [unwired: 1 in]
      n222 = Fract/Exp String To Number(string=w702) -> (number=w703:dbl[])  [unwired: 3 in, 1 out]
      n223 = Array Max & Min(array=w703) -> (max index (indices)=w699:i32)  [unwired: 3 out]
      n224 = Index Array(array=w700, index (row) #1=w699, index (col) #1=w695) -> (element #1=w698:string, element #2=w697:string)  [unwired: 2 in]
      n225 = Format Into String(format string="%s %s" ("포맷 문자열"), w698, w697) -> (resulting string=w696:string)  [unwired: 2 in, 1 out]
      n226 = Unbundle By Name(w711) -> ("추가문자열"=w710:string, "형식"=w709:string, "옵션"=w708:string)
      n227 = for {
        tunnel: w700 -> [w730] mode=indexing
        tunnel: w706 -> [w731]
        tunnel: w710 -> [w735]
        tunnel: w709 -> [w734]
        tunnel: w708 -> [w733]
        tunnel: [w729] -> w705 mode=indexing
        tunnel: w696 -> [w726]
        tunnel: [w736] -> w707 mode=indexing
        tunnel: w695 -> [w722]
        i -> [w742]
        w727 = "" ("원소")
        w717 = ""  # C4~C10
        w732 = "0"  # 엑셀문서명(C1)
        n228 = Index Array(array=w730) -> (element #1=w725:string, element #2=w720:string, element #3=w719:string, element #4=w718:string, element #5=w716:string, element #6=w715:string, element #7=w714:string, element #8=w713:string, element #9=w712:string)  [unwired: 9 in]
        n229 = Index Array(array=w730, index #2=w722) -> (element #1=w728:string, element #2=w724:string, element #3=w723:string)  [unwired: 2 in]
        n230 = String Subset(string=w731, length (rest)=5 ("길이(나머지)")) -> (substring=w737:string)  [unwired: 1 in]
        n231 = Multiply(x=w742, y=10) -> (x*y=w740:i32)
        n232 = Number To Decimal String(number=w740) -> (decimal integer string=w739:string)  [unwired: 1 in]
        n233 = Build Array(w731, w728, w727, "Angle" ("원소"), w727, w727, w724, w723) -> (w729:string[])
        n234 = Build Array(w739, w737, w731, w735, w734, w733, w725, w720, w732, w726, w719, w718, w717, w717, w717, w717, w717, w717, w716, w715, w714, w713, w712) -> (w736:string[])
      }
    }
    frame "10311-2" {
      # "9, 최대"
      n235 = Index Array(array=w743, index (row)=0 ("인덱스 (행)"), index (col)=3 ("비활성화된 인덱스 (열)")) -> (element=w746:string)
      n236 = Unbundle By Name(w765) -> ("추가문자열"=w764:string, "형식"=w763:string, "옵션"=w762:string)
      n237 = call-poly "Data Classification.vi"("인덱스"=1, "DATA 입력"=w743, "검색 문자열"="Angle_2") -> ("DATA 출력"=w744:string[][])  [unwired: 4 in, 4 out]
      n238 = Index Array(array=w744, index (col)=w751) -> (element=w750:string[])  [unwired: 1 in]
      n239 = Fract/Exp String To Number(string=w750) -> (number=w757:dbl[])  [unwired: 3 in, 1 out]
      n240 = Array Max & Min(array=w757) -> (max index (indices)=w755:i32)  [unwired: 3 out]
      n241 = Index Array(array=w744, index (row) #1=w755, index (col) #1=w751) -> (element #1=w754:string, element #2=w753:string)  [unwired: 2 in]
      n242 = Format Into String(format string="%s %s" ("포맷 문자열"), w754, w753) -> (resulting string=w752:string)  [unwired: 2 in, 1 out]
      n243 = case shown="\"mm/m\"" w746 {
        tunnel: w764 -> [_ w803]
        tunnel: w763 -> [_ w802]
        tunnel: w762 -> [_ w801]
        tunnel: [_ w800] -> w761
        tunnel: w760 -> [w766 w799]
        tunnel: [w767 w798] -> w759
        tunnel: w752 -> [w769 w797]
        tunnel: w751 -> [w768 w796]
        tunnel: w743 -> [w770 w795]
        frame Default {
          n244 = for {
            tunnel: w770 -> [w785] mode=indexing
            tunnel: [w784] -> w767 mode=indexing
            tunnel: w769 -> [_]
            tunnel: w768 -> [w782]
            tunnel: w766 -> [w774]
            w772 = "" ("원소")
            n245 = Index Array(array=w785) -> (element #2=w773:string, element #3=w776:string, element #4=w775:string)  [unwired: 9 in, 6 out]
            n246 = Index Array(array=w785, index #2=w782) -> (element #1=w783:string, element #2=w779:string, element #3=w781:string)  [unwired: 2 in]
            n247 = Fract/Exp String To Number(string=w776) -> (number=w777:dbl)  [unwired: 3 in, 1 out]
            n248 = case shown="\"Div.\"" w781 {
              selector: w781 -> [w787 _]
              tunnel: [w787 w788] -> w780
              tunnel: w779 -> [w786 w794]
              tunnel: [w786 w789] -> w778
              tunnel: w777 -> [_ w792]
              tunnel: w775 -> [_ w788]
              frame Default {
              }
              frame "Div." {
                n249 = Fract/Exp String To Number(string=w794) -> (number=w793:dbl)  [unwired: 3 in, 1 out]
                n250 = Multiply(x=w792, y=w793) -> (x*y=w791:dbl)
                n251 = Format Into String(format string="%#f" ("포맷 문자열"), w791) -> (resulting string=w789:string)  [unwired: 2 in, 1 out]
              }
            }
            n252 = Build Array(w774, w783, w773, w772, w772, w772, w778, w780) -> (w784:string[])
          }
          n253 = One Button Dialog(message="평형/각형 수준기의 감도 단위는 mm/m 로 등록 할 것.\n※ 등록완료 메시지가 나오더라도 등록되지 않음." ("메시지")) -> ()  [unwired: 1 in, 1 out]
        }
        frame "mm/m" {
          n254 = for {
            tunnel: w795 -> [w825] mode=indexing
            tunnel: w799 -> [w826]
            tunnel: w803 -> [w829]
            tunnel: w802 -> [w828]
            tunnel: w801 -> [w827]
            tunnel: [w824] -> w798 mode=indexing
            tunnel: w797 -> [w804]
            tunnel: [w830] -> w800 mode=indexing
            tunnel: w796 -> [w822]
            i -> [w836]
            w809 = "" ("원소")
            w807 = ""  # C4~C10
            w821 = "0"  # 엑셀문서명(C1)
            n255 = Index Array(array=w825, index #2=w822) -> (element #1=w823:string, element #2=w817:string, element #3=w819:string)  [unwired: 2 in]
            n256 = Index Array(array=w825) -> (element #1=w820:string, element #2=w808:string, element #3=w805:string, element #4=w806:string, element #5=w814:string, element #6=w813:string, element #7=w812:string, element #8=w811:string, element #9=w810:string)  [unwired: 9 in]
            n257 = Fract/Exp String To Number(string=w805) -> (number=w815:dbl)  [unwired: 3 in, 1 out]
            n258 = case shown="\"Div.\"" w819 {
              selector: w819 -> [w838 _]
              tunnel: [w838 w839] -> w818
              tunnel: w817 -> [w837 w845]
              tunnel: [w837 w840] -> w816
              tunnel: w815 -> [_ w843]
              tunnel: w806 -> [_ w839]
              frame Default {
              }
              frame "Div." {
                n259 = Fract/Exp String To Number(string=w845) -> (number=w844:dbl)  [unwired: 3 in, 1 out]
                n260 = Multiply(x=w843, y=w844) -> (x*y=w842:dbl)
                n261 = Format Into String(format string="%#f" ("포맷 문자열"), w842) -> (resulting string=w840:string)  [unwired: 2 in, 1 out]
              }
            }
            n262 = String Subset(string=w826, length (rest)=5 ("길이(나머지)")) -> (substring=w831:string)  [unwired: 1 in]
            n263 = Multiply(x=w836, y=10) -> (x*y=w834:i32)
            n264 = Number To Decimal String(number=w834) -> (decimal integer string=w833:string)  [unwired: 1 in]
            n265 = Build Array(w826, w823, w808, w809, w809, w809, w816, w818) -> (w824:string[])
            n266 = Build Array(w833, w831, w826, w829, w828, w827, w820, w808, w821, w804, w805, w806, w807, w807, w807, w807, w807, w807, w814, w813, w812, w811, w810) -> (w830:string[])
          }
        }
      }
    }
    frame "10404-0", "10405-0" {
      # "5, 호칭치수"
      n267 = Unbundle By Name(w854) -> ("추가문자열"=w853:string, "형식"=w852:string, "옵션"=w851:string)
      n268 = for {
        tunnel: w846 -> [w870] mode=indexing
        tunnel: w849 -> [w871]
        tunnel: w853 -> [w875]
        tunnel: w852 -> [w874]
        tunnel: w851 -> [w873]
        tunnel: [w869] -> w848 mode=indexing
        tunnel: [w876] -> w850 mode=indexing
        i -> [w882]
        w867 = "" ("원소")
        w857 = ""  # C4~C10
        w872 = "0"  # 엑셀문서명(C1)
        n269 = Index Array(array=w870) -> (element #1=w866:string, element #2=w865:string, element #3=w864:string, element #4=w856:string, element #5=w855:string)  [unwired: 5 in]
        n270 = Index Array(array=w870, index #3=3 ("인덱스")) -> (element #1=w868:string, element #2=w863:string, element #3=w861:string, element #4=w860:string)  [unwired: 3 in]
        n271 = String Subset(string=w871, length (rest)=5 ("길이(나머지)")) -> (substring=w877:string)  [unwired: 1 in]
        n272 = Multiply(x=w882, y=10) -> (x*y=w880:i32)
        n273 = Number To Decimal String(number=w880) -> (decimal integer string=w879:string)  [unwired: 1 in]
        n274 = Format Into String(format string="%s %s" ("포맷 문자열"), w856, w855) -> (resulting string=w858:string)  [unwired: 2 in, 1 out]
        n275 = Build Array(w871, w868, w863, w867, w867, w867, w861, w860) -> (w869:string[])
        n276 = Build Array(w879, w877, w871, w875, w874, w873, w866, w865, w872, w858, w864, w857, w857, w857, w857, w857, w857, w857, w856, w855, w857, w857, w857) -> (w876:string[])
      }
    }
    frame "10407-0" {
      # "7"
      n277 = Unbundle By Name(w891) -> ("추가문자열"=w890:string, "형식"=w889:string, "옵션"=w888:string)
      n278 = for {
        tunnel: w883 -> [w902] mode=indexing
        tunnel: w886 -> [w903]
        tunnel: w890 -> [w907]
        tunnel: w889 -> [w906]
        tunnel: w888 -> [w905]
        tunnel: [w901] -> w885 mode=indexing
        tunnel: [w908] -> w887 mode=indexing
        i -> [w914]
        w895 = "" ("원소")
        w896 = ""  # C7~C10
        w904 = "0"  # 엑셀문서명(C1)
        n279 = Index Array(array=w902) -> (element #1=w892:string, element #2=w900:string, element #3=w899:string, element #4=w898:string, element #5=w897:string, element #6=w893:string, element #7=w894:string)  [unwired: 7 in]
        n280 = String Subset(string=w903, length (rest)=5 ("길이(나머지)")) -> (substring=w909:string)  [unwired: 1 in]
        n281 = Multiply(x=w914, y=10) -> (x*y=w912:i32)
        n282 = Number To Decimal String(number=w912) -> (decimal integer string=w911:string)  [unwired: 1 in]
        n283 = Build Array(w903, w892, w895, w895, w895, w895, w893, w894) -> (w901:string[])
        n284 = Build Array(w911, w909, w903, w907, w906, w905, w892, w892, w904, w900, w899, w898, w897, w896, w896, w896, w896, w896, w893, w894, w896, w896, w896) -> (w908:string[])
      }
    }
    frame "10503-0" {
      # "9, 최대"
      n285 = Array Subset(array=w923, index (col)=1 ("인덱스"), length (col)=4 ("길이")) -> (w920:string[][])  [unwired: 2 in]
      n286 = call-poly "Array Deduplication.vi"("배열 in"=w920) -> ("배열 out"=w916:string[][])  [unwired: 9 in, 1 out]
      n287 = for {
        tunnel: w925 -> [w975]
        tunnel: [w974] -> w924 mode=indexing
        tunnel: w923 -> [w972]
        tunnel: w916 -> [w971] mode=indexing
        n288 = for {
          shift-right: [w986] -> w973
          shift-left: w972 -> [w985]
          tunnel: w971 -> [w984] mode=indexing
          i -> [w983]
          n289 = Increment(x=w983) -> (x+1=w982:i32)
          n290 = call-poly "Data Classification.vi"("인덱스"=w982, "DATA 입력"=w985, "검색 문자열"=w984) -> ("DATA 출력"=w986:string[][])  [unwired: 4 in, 4 out]
        }
        n291 = Index Array(array=w973, index (col)=w975) -> (element=w980:string[])  [unwired: 1 in]
        n292 = Fract/Exp String To Number(string=w980) -> (number=w981:dbl[])  [unwired: 3 in, 1 out]
        n293 = Array Max & Min(array=w981) -> (max index (indices)=w979:i32)  [unwired: 3 out]
        n294 = Index Array(array=w973, index (row) #1=w979, index (col) #1=w975) -> (element #1=w978:string, element #2=w976:string)  [unwired: 2 in]
        n295 = Format Into String(format string="%s %s" ("포맷 문자열"), w978, w976) -> (resulting string=w974:string)  [unwired: 2 in, 1 out]
      }
      n296 = Unbundle By Name(w929) -> ("추가문자열"=w919:string, "형식"=w918:string, "옵션"=w917:string)
      n297 = for {
        tunnel: w923 -> [w951] mode=indexing
        tunnel: w927 -> [w952]
        tunnel: w919 -> [w958]
        tunnel: w918 -> [w957]
        tunnel: w917 -> [w956]
        tunnel: [w950] -> w915 mode=indexing
        tunnel: [w961] -> w928 mode=indexing
        tunnel: w924 -> [w938]
        tunnel: w916 -> [w936]
        i -> [w965]
        w949 = ""
        w953 = ""  # C6~C10
        w954 = "0"  # 엑셀문서명(C1)
        n298 = Index Array(array=w951) -> (element #1=w955:string, element #2=w935:string, element #3=w934:string, element #4=w933:string, element #5=w932:string, element #6=w943:string, element #7=w942:string, element #8=w941:string, element #9=w940:string, element #10=w939:string)  [unwired: 10 in]
        n299 = Index Array(array=w951) -> (element #1=w944:string, element #3=w948:string, element #4=w947:string, element #5=w946:string, element #6=w945:string)  [unwired: 6 in, 1 out]
        n300 = String Subset(string=w952, length (rest)=5 ("길이(나머지)")) -> (substring=w960:string)  [unwired: 1 in]
        n301 = Build Array(w935, w934, w933, w932) -> (w931:string[])
        n302 = Multiply(x=w965, y=10) -> (x*y=w963:i32)
        n303 = for {
          tunnel: w936 -> [w969] mode=indexing
          tunnel: w931 -> [w970]
          tunnel: [w966] -> w930
          i -> [w966]
          stop <- w967 stop-if-true
          n304 = Equal?(x=w970, y=w969) -> (x = y?=w968:bool[])
          n305 = And Array Elements(Boolean array=w968) -> (logical AND=w967:bool)
        }
        n306 = Number To Decimal String(number=w963) -> (decimal integer string=w959:string)  [unwired: 1 in]
        n307 = Index Array(array=w938, index=w930) -> (element=w937:string)
        n308 = Build Array(w952, w944, w949, w949, w948, w947, w946, w945) -> (w950:string[])
        n309 = Build Array(w959, w960, w952, w958, w957, w956, w955, w935, w954, w937, w934, w933, w932, w953, w953, w953, w953, w953, w943, w942, w941, w940, w939) -> (w961:string[])
      }
    }
    frame "10504-1", "10511-1", "10511-2", "20411-1", "20411-4", "20412-1", "20412-2" {
      w988 = 1 ("비활성화된 인덱스 (열)")
      # "7, 최대, 최소"
      n310 = Index Array(array=w995, index (col)=w988) -> (element=w996:string[])  [unwired: 1 in]
      n311 = Increment(x=w988) -> (x+1=w987:i32)
      n312 = call-poly "Array Deduplication.vi"("배열 in"=w996) -> ("배열 out"=w994:string[])  [unwired: 9 in, 1 out]
      n313 = for {
        tunnel: w995 -> [w1014]
        tunnel: w994 -> [w1013] mode=indexing
        tunnel: [w1003] -> w993 mode=indexing
        tunnel: w988 -> [w1002]
        tunnel: w987 -> [w1001]
        n314 = call "Data Class_2D Str.vi"("인덱스"=w1002, "DATA 입력"=w1014, "검색 문자열"=w1013) -> ("DATA 출력"=w1010:string[][])  [unwired: 4 in, 4 out]
        n315 = Index Array(array=w1010, index (col)=w1001) -> (element=w1012:string[])  [unwired: 1 in]
        n316 = Fract/Exp String To Number(string=w1012) -> (number=w1011:dbl[])  [unwired: 3 in, 1 out]
        n317 = Array Max & Min(array=w1011) -> (max index (indices)=w1009:i32)  [unwired: 3 out]
        n318 = Index Array(array=w1010, index (row) #1=w1009, index (col) #1=w1002) -> (element #1=w1005:string, element #2=w1007:string, element #3=w1006:string)  [unwired: 4 in]
        n319 = Format Into String(format string="%s %s" ("포맷 문자열"), w1007, w1006) -> (resulting string=w1004:string)  [unwired: 2 in, 1 out]
        n320 = Build Array(w1005, w1004) -> (w1003:string[])
      }
      n321 = Unbundle By Name(w1000) -> ("추가문자열"=w999:string, "형식"=w998:string, "옵션"=w997:string)
      n322 = for {
        tunnel: w995 -> [w1020] mode=indexing
        tunnel: w991 -> [w1021]
        tunnel: w999 -> [w1039]
        tunnel: w998 -> [w1038]
        tunnel: w997 -> [w1037]
        tunnel: [w1019] -> w990 mode=indexing
        tunnel: w993 -> [w1028]
        tunnel: [w1040] -> w992 mode=indexing
        i -> [w1046]
        w1015 = "" ("원소")
        w1031 = ""  # C3~C10
        w1035 = "0"  # 엑셀문서명(C1)
        n323 = Index Array(array=w1020) -> (element #1=w1036:string, element #2=w1032:string, element #3=w1026:string, element #4=w1025:string, element #5=w1024:string, element #6=w1023:string, element #7=w1022:string)  [unwired: 7 in]
        n324 = Index Array(array=w1020) -> (element #1=w1018:string, element #3=w1017:string, element #4=w1016:string)  [unwired: 4 in, 1 out]
        n325 = String Subset(string=w1021, length (rest)=5 ("길이(나머지)")) -> (substring=w1041:string)  [unwired: 1 in]
        n326 = Index Array(array=w1028, index (col)=0 ("비활성화된 인덱스 (열)")) -> (element=w1033:string[])  [unwired: 1 in]
        n327 = Multiply(x=w1046, y=10) -> (x*y=w1044:i32)
        n328 = Search 1D Array(1D array=w1033, element=w1032) -> (index of element=w1030:i32)  [unwired: 1 in]
        n329 = Number To Decimal String(number=w1044) -> (decimal integer string=w1043:string)  [unwired: 1 in]
        n330 = Index Array(array=w1028, index (row)=w1030, index (col)=1 ("비활성화된 인덱스 (열)")) -> (element=w1027:string)
        n331 = Build Array(w1021, w1018, w1015, w1015, w1015, w1015, w1017, w1016) -> (w1019:string[])
        n332 = Build Array(w1043, w1041, w1021, w1039, w1038, w1037, w1036, w1032, w1035, w1027, w1031, w1031, w1031, w1031, w1031, w1031, w1031, w1031, w1026, w1025, w1024, w1023, w1022) -> (w1040:string[])
      }
    }
    frame "10517-0" {
      w1047 = 1 ("비활성화된 인덱스 (열)")
      # "8, 최대"
      n333 = Index Array(array=w1050, index (col)=w1047) -> (element=w1049:string[])  [unwired: 1 in]
      n334 = call-poly "Array Deduplication.vi"("배열 in"=w1049) -> ("배열 out"=w1048:string[])  [unwired: 9 in, 1 out]
      n335 = for {
        tunnel: [w1067] -> w1052 mode=indexing
        tunnel: w1051 -> [w1062]
        tunnel: w1050 -> [w1066]
        tunnel: w1048 -> [w1064] mode=indexing
        tunnel: w1047 -> [w1065]
        n336 = call-poly "Data Classification.vi"("인덱스"=w1065, "DATA 입력"=w1066, "검색 문자열"=w1064) -> ("DATA 출력"=w1063:string[][])  [unwired: 4 in, 4 out]
        n337 = Index Array(array=w1063, index (col)=w1062) -> (element=w1061:string[])  [unwired: 1 in]
        n338 = Fract/Exp String To Number(string=w1061) -> (number=w1073:dbl[])  [unwired: 3 in, 1 out]
        n339 = Array Max & Min(array=w1073) -> (max index (indices)=w1071:i32)  [unwired: 3 out]
        n340 = Index Array(array=w1063, index (row) #1=w1071, index (col) #1=w1062) -> (element #1=w1070:string, element #2=w1069:string)  [unwired: 2 in]
        n341 = Format Into String(format string="%s %s" ("포맷 문자열"), w1070, w1069) -> (resulting string=w1068:string)  [unwired: 2 in, 1 out]
        n342 = Build Array(w1064, w1068) -> (w1067:string[])
      }
      n343 = Unbundle By Name(w1060) -> ("추가문자열"=w1059:string, "형식"=w1058:string, "옵션"=w1057:string)
      n344 = for {
        tunnel: w1050 -> [w1095] mode=indexing
        tunnel: w1055 -> [w1096]
        tunnel: w1059 -> [w1100]
        tunnel: w1058 -> [w1099]
        tunnel: w1057 -> [w1098]
        tunnel: [w1094] -> w1054 mode=indexing
        tunnel: w1052 -> [w1080]
        tunnel: [w1101] -> w1056 mode=indexing
        i -> [w1107]
        w1091 = "" ("원소")
        w1087 = ""  # C4~C10
        w1097 = "0"  # 엑셀문서명(C1)
        n345 = Index Array(array=w1095) -> (element #1=w1090:string, element #2=w1078:string, element #3=w1086:string, element #4=w1085:string, element #5=w1084:string, element #6=w1083:string, element #7=w1082:string, element #8=w1081:string)  [unwired: 8 in]
        n346 = Index Array(array=w1095) -> (element #1=w1089:string, element #2=w1088:string, element #3=w1093:string, element #4=w1092:string)  [unwired: 4 in]
        n347 = String Subset(string=w1096, length (rest)=5 ("길이(나머지)")) -> (substring=w1102:string)  [unwired: 1 in]
        n348 = Index Array(array=w1080, index (col) #1=0 ("비활성화된 인덱스 (열)")) -> (element #1=w1079:string[], element #2=w1077:string[])  [unwired: 3 in]
        n349 = Multiply(x=w1107, y=10) -> (x*y=w1105:i32)
        n350 = Number To Decimal String(number=w1105) -> (decimal integer string=w1104:string)  [unwired: 1 in]
        n351 = Search 1D Array(1D array=w1079, element=w1078) -> (index of element=w1076:i32)  [unwired: 1 in]
        n352 = Index Array(array=w1077, index=w1076) -> (element=w1075:string)
        n353 = Build Array(w1096, w1089, w1088, w1091, w1091, w1091, w1093, w1092) -> (w1094:string[])
        n354 = Build Array(w1104, w1102, w1096, w1100, w1099, w1098, w1090, w1078, w1097, w1075, w1086, w1087, w1087, w1087, w1087, w1087, w1087, w1087, w1085, w1084, w1083, w1082, w1081) -> (w1101:string[])
      }
    }
    frame "10601-1", "10609-1" {
      # "7, 최대"
      n355 = Index Array(array=w1109, index (col)=w1108) -> (element=w1115:string[])  [unwired: 1 in]
      n356 = Fract/Exp String To Number(string=w1115) -> (number=w1116:dbl[])  [unwired: 3 in, 1 out]
      n357 = Array Max & Min(array=w1116) -> (max index (indices)=w1113:i32)  [unwired: 3 out]
      n358 = Index Array(array=w1109, index (row) #1=w1113, index (col) #1=w1108) -> (element #1=w1112:string, element #2=w1111:string)  [unwired: 2 in]
      n359 = Format Into String(format string="%s %s" ("포맷 문자열"), w1112, w1111) -> (resulting string=w1110:string)  [unwired: 2 in, 1 out]
      n360 = Unbundle By Name(w1124) -> ("추가문자열"=w1123:string, "형식"=w1122:string, "옵션"=w1121:string)
      n361 = for {
        tunnel: w1109 -> [w1135] mode=indexing
        tunnel: w1119 -> [w1136]
        tunnel: w1123 -> [w1145]
        tunnel: w1122 -> [w1144]
        tunnel: w1121 -> [w1143]
        tunnel: [w1134] -> w1118 mode=indexing
        tunnel: w1110 -> [w1132]
        tunnel: [w1146] -> w1120 mode=indexing
        tunnel: w1108 -> [w1126]
        i -> [w1152]
        w1133 = "" ("원소")
        w1131 = ""  # C4~C10
        w1142 = "0"  # 엑셀문서명(C1)
        n362 = Index Array(array=w1135) -> (element #1=w1128:string, element #2=w1127:string, element #3=w1141:string, element #4=w1140:string, element #5=w1139:string, element #6=w1138:string, element #7=w1137:string)  [unwired: 7 in]
        n363 = Index Array(array=w1135, index #3=w1126) -> (element #1=w1125:string, element #3=w1130:string, element #4=w1129:string)  [unwired: 3 in, 1 out]
        n364 = String Subset(string=w1136, length (rest)=5 ("길이(나머지)")) -> (substring=w1147:string)  [unwired: 1 in]
        n365 = Multiply(x=w1152, y=10) -> (x*y=w1150:i32)
        n366 = Number To Decimal String(number=w1150) -> (decimal integer string=w1149:string)  [unwired: 1 in]
        n367 = Build Array(w1136, w1125, w1133, w1133, w1133, w1133, w1130, w1129) -> (w1134:string[])
        n368 = Build Array(w1149, w1147, w1136, w1145, w1144, w1143, w1128, w1128, w1142, w1132, w1127, w1131, w1131, w1131, w1131, w1131, w1131, w1131, w1141, w1140, w1139, w1138, w1137) -> (w1146:string[])
      }
    }
    frame "20109-0" {
      w1154 = 1 ("비활성화된 인덱스 (열)")
      n369 = Index Array(array=w1161, index (col)=w1154) -> (element=w1162:string[])  [unwired: 1 in]
      n370 = Increment(x=w1154) -> (x+1=w1153:i32)
      n371 = call-poly "Array Deduplication.vi"("배열 in"=w1162) -> ("배열 out"=w1160:string[])  [unwired: 9 in, 1 out]
      n372 = for {
        tunnel: w1161 -> [w1180]
        tunnel: w1160 -> [w1179] mode=indexing
        tunnel: [w1169] -> w1159 mode=indexing
        tunnel: w1154 -> [w1168]
        tunnel: w1153 -> [w1167]
        n373 = call "Data Class_2D Str.vi"("인덱스"=w1168, "DATA 입력"=w1180, "검색 문자열"=w1179) -> ("DATA 출력"=w1176:string[][])  [unwired: 4 in, 4 out]
        n374 = Index Array(array=w1176, index (col)=w1167) -> (element=w1178:string[])  [unwired: 1 in]
        n375 = Fract/Exp String To Number(string=w1178) -> (number=w1177:dbl[])  [unwired: 3 in, 1 out]
        n376 = Array Max & Min(array=w1177) -> (max index (indices)=w1175:i32)  [unwired: 3 out]
        n377 = Index Array(array=w1176, index (row) #1=w1175, index (col) #1=w1168) -> (element #1=w1171:string, element #2=w1173:string, element #3=w1172:string)  [unwired: 4 in]
        n378 = Format Into String(format string="%s %s" ("포맷 문자열"), w1173, w1172) -> (resulting string=w1170:string)  [unwired: 2 in, 1 out]
        n379 = Build Array(w1171, w1170) -> (w1169:string[])
      }
      n380 = Unbundle By Name(w1166) -> ("추가문자열"=w1165:string, "형식"=w1164:string, "옵션"=w1163:string)
      n381 = for {
        tunnel: w1161 -> [w1187] mode=indexing
        tunnel: w1157 -> [w1188]
        tunnel: w1165 -> [w1206]
        tunnel: w1164 -> [w1205]
        tunnel: w1163 -> [w1204]
        tunnel: [w1184] -> w1156 mode=indexing
        tunnel: w1159 -> [w1190]
        tunnel: [w1207] -> w1158 mode=indexing
        i -> [w1213]
        w1181 = "" ("원소")
        w1198 = ""  # C3~C10
        w1202 = "0"  # 엑셀문서명(C1)
        n382 = Index Array(array=w1187) -> (element #1=w1203:string, element #2=w1199:string, element #3=w1197:string, element #4=w1196:string, element #5=w1194:string, element #6=w1193:string)  [unwired: 6 in]
        n383 = Index Array(array=w1187) -> (element #1=w1186:string, element #2=w1185:string, element #3=w1183:string, element #4=w1182:string)  [unwired: 4 in]
        n384 = String Subset(string=w1188, length (rest)=5 ("길이(나머지)")) -> (substring=w1208:string)  [unwired: 1 in]
        n385 = Index Array(array=w1190, index (col)=0 ("비활성화된 인덱스 (열)")) -> (element=w1200:string[])  [unwired: 1 in]
        n386 = Multiply(x=w1213, y=10) -> (x*y=w1211:i32)
        n387 = Search 1D Array(1D array=w1200, element=w1199) -> (index of element=w1192:i32)  [unwired: 1 in]
        n388 = Number To Decimal String(number=w1211) -> (decimal integer string=w1210:string)  [unwired: 1 in]
        n389 = Index Array(array=w1190, index (row)=w1192, index (col)=1 ("비활성화된 인덱스 (열)")) -> (element=w1189:string)
        n390 = Build Array(w1188, w1186, w1185, w1181, w1181, w1181, w1183, w1182) -> (w1184:string[])
        n391 = Build Array(w1210, w1208, w1188, w1206, w1205, w1204, w1203, w1199, w1202, w1189, w1198, w1198, w1198, w1198, w1198, w1198, w1198, w1198, w1197, w1196, "Digital" ("원소"), w1194, w1193) -> (w1207:string[])
      }
    }
    frame "20116-1" {
      # "5, 없음"
      n392 = Unbundle By Name(w1222) -> ("추가문자열"=w1221:string, "형식"=w1220:string, "옵션"=w1219:string)
      n393 = for {
        tunnel: w1218 -> [w1228] mode=indexing
        tunnel: w1216 -> [w1230]
        tunnel: w1221 -> [w1240]
        tunnel: w1220 -> [w1239]
        tunnel: w1219 -> [w1238]
        tunnel: [w1229] -> w1215 mode=indexing
        tunnel: [w1241] -> w1217 mode=indexing
        i -> [w1247]
        w1225 = "" ("원소")
        w1231 = ""  # C3~C10
        w1236 = "0"  # 엑셀문서명(C1)
        n394 = Index Array(array=w1228) -> (element #1=w1237:string, element #2=w1235:string, element #3=w1234:string, element #4=w1233:string, element #5=w1232:string)  [unwired: 5 in]
        n395 = Index Array(array=w1228, index #2=3 ("인덱스")) -> (element #1=w1223:string, element #2=w1227:string, element #3=w1226:string)  [unwired: 2 in]
        n396 = String Subset(string=w1230, length (rest)=5 ("길이(나머지)")) -> (substring=w1242:string)  [unwired: 1 in]
        n397 = Multiply(x=w1247, y=10) -> (x*y=w1245:i32)
        n398 = Number To Decimal String(number=w1245) -> (decimal integer string=w1244:string)  [unwired: 1 in]
        n399 = Build Array(w1230, w1223, w1225, w1225, w1225, w1225, w1227, w1226) -> (w1229:string[])
        n400 = Build Array(w1244, w1242, w1230, w1240, w1239, w1238, w1237, w1235, w1236, w1234, w1231, w1231, w1231, w1231, w1231, w1231, w1231, w1231, w1233, w1232, w1231, w1231, w1231) -> (w1241:string[])
      }
    }
    frame "20116-2" {
      # "8, 없음"
      n401 = Unbundle By Name(w1256) -> ("추가문자열"=w1255:string, "형식"=w1254:string, "옵션"=w1253:string)
      n402 = for {
        tunnel: w1252 -> [w1268] mode=indexing
        tunnel: w1250 -> [w1270]
        tunnel: w1255 -> [w1277]
        tunnel: w1254 -> [w1276]
        tunnel: w1253 -> [w1275]
        tunnel: [w1269] -> w1249 mode=indexing
        tunnel: [w1278] -> w1251 mode=indexing
        i -> [w1284]
        w1257 = "" ("원소")
        w1258 = ""  # C6~C10
        w1273 = "0"  # 엑셀문서명(C1)
        n403 = Index Array(array=w1268) -> (element #1=w1274:string, element #2=w1272:string, element #3=w1271:string, element #4=w1263:string, element #5=w1262:string, element #6=w1261:string, element #7=w1259:string, element #8=w1260:string)  [unwired: 8 in]
        n404 = Index Array(array=w1268, index #2=6 ("인덱스")) -> (element #1=w1267:string, element #2=w1266:string, element #3=w1265:string)  [unwired: 2 in]
        n405 = String Subset(string=w1270, length (rest)=5 ("길이(나머지)")) -> (substring=w1279:string)  [unwired: 1 in]
        n406 = Multiply(x=w1284, y=10) -> (x*y=w1282:i32)
        n407 = Number To Decimal String(number=w1282) -> (decimal integer string=w1281:string)  [unwired: 1 in]
        n408 = Build Array(w1270, w1267, w1257, w1257, w1257, w1257, w1266, w1265) -> (w1269:string[])
        n409 = Build Array(w1281, w1279, w1270, w1277, w1276, w1275, w1274, w1272, w1273, w1271, w1263, w1262, w1261, w1258, w1258, w1258, w1258, w1258, w1259, w1260, w1258, w1258, w1258) -> (w1278:string[])
      }
    }
    frame "20202-0" {
      w1305 = 0 ("비활성화된 인덱스 (열)")
      n410 = Index Array(array=w1297, index (row) #1=0 ("인덱스 (행)"), index (col) #1=2 ("비활성화된 인덱스 (열)")) -> (element #1=w1293:string, element #2=w1292:string)  [unwired: 2 in]
      n411 = Index Array(array=w1297, index (col)=w1305) -> (element=w1312:string[])  [unwired: 1 in]
      n412 = call-poly "Array Deduplication.vi"("배열 in"=w1312) -> ("배열 out"=w1311:string[])  [unwired: 9 in, 1 out]
      n413 = for {
        tunnel: w1297 -> [w1389] mode=indexing
        tunnel: [w1392] -> w1304 mode=indexing
        tunnel: [w1391] -> w1302
        tunnel: [w1390] -> w1301
        tunnel: w1293 -> [w1387]
        tunnel: w1292 -> [w1386]
        tunnel: [w1385] -> w1291 mode=indexing
        n414 = Index Array(array=w1389, index #1=4 ("인덱스")) -> (element #1=w1394:string, element #2=w1391:string)  [unwired: 1 in]
        n415 = Replace Array Subset(array=w1389, new element #1=w1387, index #1=2 ("인덱스"), new element #2=w1386) -> (w1385:string[])  [unwired: 1 in]
        n416 = call "Unit Conversion.vi"("환산단위"="kN", "입력단위"=w1391, "입력값"=w1394) -> ("환산단위"=w1390:string, "환산값 (DBL)"=w1392:dbl)  [unwired: 3 in, 4 out]
      }
      n417 = Unbundle By Name(w1316) -> ("추가문자열"=w1315:string, "형식"=w1314:string, "옵션"=w1313:string)
      n418 = for {
        tunnel: w1297 -> [w1409]
        tunnel: w1311 -> [w1408] mode=indexing
        tunnel: [w1401] -> w1310 mode=indexing
        tunnel: w1305 -> [w1400]
        w1399 = 4 ("비활성화된 인덱스 (열)")
        n419 = call "Data Class_2D Str.vi"("인덱스"=w1400, "DATA 입력"=w1409, "검색 문자열"=w1408) -> ("DATA 출력"=w1405:string[][])  [unwired: 4 in, 4 out]
        n420 = Index Array(array=w1405, index (col)=w1399) -> (element=w1407:string[])  [unwired: 1 in]
        n421 = Fract/Exp String To Number(string=w1407) -> (number=w1406:dbl[])  [unwired: 3 in, 1 out]
        n422 = Array Max & Min(array=w1406) -> (max index (indices)=w1398:i32)  [unwired: 3 out]
        n423 = Index Array(array=w1405, index (row) #1=w1398, index (col) #1=w1400, index (row) #2=w1398, index (col) #2=w1399) -> (element #1=w1403:string, element #2=w1397:string, element #3=w1396:string)  [unwired: 2 in]
        n424 = Format Into String(format string="%s %s" ("포맷 문자열"), w1397, w1396) -> (resulting string=w1402:string)  [unwired: 2 in, 1 out]
        n425 = Build Array(w1403, w1402) -> (w1401:string[])
      }
      n426 = call "Unit Conversion.vi"("환산단위"="kN", "입력단위"=w1292, "입력값"=w1293) -> ("환산값 (DBL)"=w1290:dbl)  [unwired: 3 in, 5 out]
      n427 = Multiply(x=w1290, y=1.1) -> (x*y=w1287:dbl)
      n428 = Array Max & Min(array=w1304) -> (max value=w1288:dbl)  [unwired: 3 out]
      n429 = Not Equal?(x=w1302, y=w1301) -> (x != y?=w1300:bool)
      n430 = Less Or Equal?(x=w1287, y=w1288) -> (x <= y?=w1286:bool)
      n431 = Less Or Equal?(x=w1288, y=5.0) -> (x <= y?=w1299:bool)
      n432 = Compound Arithmetic op=AND(w1299, w1300) -> (w1298:bool)
      n433 = Or(x=w1286, y=w1298) -> (x .or. y?=w1285:bool)
      n434 = case shown="참" w1285 {
        tunnel: w1315 -> [_ w1344]
        tunnel: w1314 -> [_ w1343]
        tunnel: w1313 -> [_ w1342]
        tunnel: w1310 -> [_ w1341]
        tunnel: [_ w1340] -> w1309
        tunnel: w1308 -> [w1323 w1339]
        tunnel: [w1322 w1338] -> w1307
        tunnel: w1291 -> [w1321 w1337]
        tunnel: w1286 -> [w1319 _]
        frame True {
          n435 = for {
            tunnel: w1321 -> [w1336] mode=indexing
            tunnel: w1323 -> [w1335]
            tunnel: [w1334] -> w1322 mode=indexing
            w1324 = "0" ("원소")
            n436 = Index Array(array=w1336, index #2=3 ("인덱스")) -> (element #1=w1328:string, element #2=w1327:string, element #3=w1326:string)  [unwired: 2 in]
            n437 = Not Equal?(x=w1327, y="0") -> (x != y?=w1329:bool)
            n438 = Select(t=w1327, s=w1329, f="0.5" ("t")) -> ()  [unwired: 1 out]
            n439 = Select(t=w1326, s=w1329, f="kN" ("t")) -> (s? t:f=w1330:string)
            n440 = Build Array(w1335, w1328, w1324, w1324, w1324, w1324, w1324, w1330) -> (w1334:string[])
          }
          n441 = Select(t="포함된 교정점이 장비 최대용량의 110% 보다 큼. 장비파손의 우려가 있음.\n※ 등록완료 메시지가 나오더라도 등록되지 않음." ("메시지"), s=w1319, f="5 kN 이하 장비는 교정점과 단위를 실하중 힘 교정기 기준으로 등록 할 것.\n(최소 0.05 kN 간격, kN 단위)\n※ 등록완료 메시지가 나오더라도 등록되지 않음." ("메시지")) -> (s? t:f=w1317:string)
          n442 = One Button Dialog(message=w1317) -> ()  [unwired: 1 in, 1 out]
        }
        frame False {
          n443 = for {
            tunnel: w1337 -> [w1368] mode=indexing
            tunnel: w1339 -> [w1367]
            tunnel: w1344 -> [w1377]
            tunnel: w1343 -> [w1376]
            tunnel: w1342 -> [w1375]
            tunnel: [w1366] -> w1338 mode=indexing
            tunnel: w1341 -> [w1369]
            tunnel: [w1378] -> w1340 mode=indexing
            i -> [w1384]
            w1355 = "" ("원소")
            w1351 = ""  # C4~C10
            w1374 = "0"  # 엑셀문서명(C1)
            n444 = Index Array(array=w1368) -> (element #1=w1353:string, element #2=w1354:string, element #3=w1346:string, element #4=w1345:string, element #5=w1347:string, element #6=w1348:string, element #7=w1349:string, element #8=w1350:string)  [unwired: 8 in]
            n445 = Index Array(array=w1368, index #2=4 ("인덱스")) -> (element #1=w1359:string, element #2=w1357:string, element #3=w1356:string)  [unwired: 2 in]
            n446 = String Subset(string=w1367, length (rest)=5 ("길이(나머지)")) -> (substring=w1379:string)  [unwired: 1 in]
            n447 = Index Array(array=w1369, index (col)=0 ("비활성화된 인덱스 (열)")) -> (element=w1372:string[])  [unwired: 1 in]
            n448 = Multiply(x=w1384, y=10) -> (x*y=w1382:i32)
            n449 = Not Equal?(x=w1357, y="0") -> (x != y?=w1360:bool)
            n450 = Number To Decimal String(number=w1382) -> (decimal integer string=w1381:string)  [unwired: 1 in]
            n451 = Search 1D Array(1D array=w1372, element=w1353) -> (index of element=w1371:i32)  [unwired: 1 in]
            n452 = Index Array(array=w1369, index (row)=w1371, index (col)=1 ("비활성화된 인덱스 (열)")) -> (element=w1358:string)
            n453 = Select(t=w1357, s=w1360, f="0.5" ("t")) -> (s? t:f=w1363:string)
            n454 = Select(t=w1356, s=w1360, f="kN" ("t")) -> (s? t:f=w1361:string)
            n455 = Build Array(w1367, w1359, w1355, w1355, w1355, w1355, w1363, w1361) -> (w1366:string[])
            n456 = Build Array(w1381, w1379, w1367, w1377, w1376, w1375, w1353, w1354, w1374, w1358, w1346, w1345, w1351, w1351, w1351, w1351, w1351, w1351, w1347, w1348, w1349, w1350, w1348) -> (w1378:string[])
          }
        }
      }
    }
    frame "20204-0" {
      w1410 = 0 ("비활성화된 인덱스 (열)")
      n457 = Index Array(array=w1417, index (col)=w1410) -> (element=w1418:string[])  [unwired: 1 in]
      n458 = call-poly "Array Deduplication.vi"("배열 in"=w1418) -> ("배열 out"=w1416:string[])  [unwired: 9 in, 1 out]
      n459 = for {
        tunnel: w1417 -> [w1436]
        tunnel: w1416 -> [w1435] mode=indexing
        tunnel: [w1427] -> w1415 mode=indexing
        tunnel: w1410 -> [w1426]
        n460 = call "Data Class_2D Str.vi"("인덱스"=w1426, "DATA 입력"=w1436, "검색 문자열"=w1435) -> ("DATA 출력"=w1432:string[][])  [unwired: 4 in, 4 out]
        n461 = Index Array(array=w1432, index (col)=3 ("비활성화된 인덱스 (열)")) -> (element=w1434:string[])  [unwired: 1 in]
        n462 = Fract/Exp String To Number(string=w1434) -> (number=w1433:dbl[])  [unwired: 3 in, 1 out]
        n463 = Array Max & Min(array=w1433) -> (max index (indices)=w1431:i32)  [unwired: 3 out]
        n464 = Index Array(array=w1432, index (row) #1=w1431, index (col) #1=w1426) -> (element #1=w1429:string, element #4=w1423:string, element #5=w1424:string)  [unwired: 8 in, 2 out]
        n465 = Format Into String(format string="%s %s" ("포맷 문자열"), w1423, w1424) -> (resulting string=w1428:string)  [unwired: 2 in, 1 out]
        n466 = Build Array(w1429, w1428) -> (w1427:string[])
      }
      n467 = Unbundle By Name(w1422) -> ("추가문자열"=w1421:string, "형식"=w1420:string, "옵션"=w1419:string)
      n468 = for {
        tunnel: w1417 -> [w1459] mode=indexing
        tunnel: w1413 -> [w1458]
        tunnel: w1421 -> [w1469]
        tunnel: w1420 -> [w1468]
        tunnel: w1419 -> [w1467]
        tunnel: [w1457] -> w1412 mode=indexing
        tunnel: w1415 -> [w1461]
        tunnel: [w1470] -> w1414 mode=indexing
        i -> [w1476]
        w1437 = "" ("원소")
        w1454 = ""  # C4~C10
        w1466 = "0"  # 엑셀문서명(C1)
        n469 = Index Array(array=w1459) -> (element #1=w1460:string, element #2=w1448:string, element #3=w1446:string, element #4=w1445:string, element #5=w1444:string, element #6=w1443:string, element #7=w1442:string, element #8=w1441:string)  [unwired: 8 in]
        n470 = Index Array(array=w1459, index #2=3 ("인덱스")) -> (element #1=w1449:string, element #2=w1440:string, element #3=w1439:string)  [unwired: 2 in]
        n471 = String Subset(string=w1458, length (rest)=5 ("길이(나머지)")) -> (substring=w1471:string)  [unwired: 1 in]
        n472 = Index Array(array=w1461, index (col)=0 ("비활성화된 인덱스 (열)")) -> (element=w1464:string[])  [unwired: 1 in]
        n473 = Multiply(x=w1476, y=10) -> (x*y=w1474:i32)
        n474 = Not Equal?(x=w1440, y="0") -> (x != y?=w1450:bool)
        n475 = Number To Decimal String(number=w1474) -> (decimal integer string=w1473:string)  [unwired: 1 in]
        n476 = Search 1D Array(1D array=w1464, element=w1460) -> (index of element=w1463:i32)  [unwired: 1 in]
        n477 = Index Array(array=w1461, index (row)=w1463, index (col)=1 ("비활성화된 인덱스 (열)")) -> (element=w1447:string)
        n478 = Select(t=w1440, s=w1450, f="0.2" ("t")) -> (s? t:f=w1453:string)
        n479 = Select(t=w1439, s=w1450, f="N" ("t")) -> (s? t:f=w1451:string)
        n480 = Build Array(w1458, w1449, w1437, w1437, w1437, w1437, w1453, w1451) -> (w1457:string[])
        n481 = Build Array(w1473, w1471, w1458, w1469, w1468, w1467, w1460, w1448, w1466, w1447, w1446, w1454, w1454, w1454, w1454, w1454, w1454, w1454, w1445, w1444, w1443, w1442, w1441) -> (w1470:string[])
      }
    }
    frame "20302-0" {
      w1478 = 0 ("비활성화된 인덱스 (열)")
      n482 = Index Array(array=w1485, index (col)=w1478) -> (element=w1486:string[])  [unwired: 1 in]
      n483 = Increment(x=w1478) -> (x+1=w1477:i32)
      n484 = call-poly "Array Deduplication.vi"("배열 in"=w1486) -> ("배열 out"=w1484:string[])  [unwired: 9 in, 1 out]
      n485 = for {
        tunnel: w1485 -> [w1504]
        tunnel: w1484 -> [w1503] mode=indexing
        tunnel: [w1493] -> w1483 mode=indexing
        tunnel: w1478 -> [w1492]
        tunnel: w1477 -> [w1491]
        n486 = call "Data Class_2D Str.vi"("인덱스"=w1492, "DATA 입력"=w1504, "검색 문자열"=w1503) -> ("DATA 출력"=w1500:string[][])  [unwired: 4 in, 4 out]
        n487 = Index Array(array=w1500, index (col)=w1491) -> (element=w1502:string[])  [unwired: 1 in]
        n488 = Fract/Exp String To Number(string=w1502) -> (number=w1501:dbl[])  [unwired: 3 in, 1 out]
        n489 = Array Max & Min(array=w1501) -> (max index (indices)=w1499:i32)  [unwired: 3 out]
        n490 = Index Array(array=w1500, index (row) #1=w1499, index (col) #1=w1492) -> (element #1=w1495:string, element #2=w1497:string, element #3=w1496:string)  [unwired: 4 in]
        n491 = Format Into String(format string="%s %s" ("포맷 문자열"), w1497, w1496) -> (resulting string=w1494:string)  [unwired: 2 in, 1 out]
        n492 = Build Array(w1495, w1494) -> (w1493:string[])
      }
      n493 = Unbundle By Name(w1490) -> ("추가문자열"=w1489:string, "형식"=w1488:string, "옵션"=w1487:string)
      n494 = for {
        tunnel: w1485 -> [w1518] mode=indexing
        tunnel: w1481 -> [w1516]
        tunnel: w1489 -> [w1534]
        tunnel: w1488 -> [w1533]
        tunnel: w1487 -> [w1532]
        tunnel: [w1515] -> w1480 mode=indexing
        tunnel: w1483 -> [w1526]
        tunnel: [w1535] -> w1482 mode=indexing
        i -> [w1541]
        w1505 = "" ("원소")
        w1510 = ""  # C3~C10
        w1531 = "0"  # 엑셀문서명(C1)
        n495 = Index Array(array=w1518) -> (element #1=w1524:string, element #2=w1523:string, element #3=w1522:string, element #4=w1521:string, element #5=w1520:string, element #6=w1519:string)  [unwired: 6 in]
        n496 = Index Array(array=w1518) -> (element #1=w1517:string, element #2=w1511:string, element #3=w1509:string)  [unwired: 3 in]
        n497 = String Subset(string=w1516, length (rest)=5 ("길이(나머지)")) -> (substring=w1536:string)  [unwired: 1 in]
        n498 = Index Array(array=w1526, index (col)=0 ("비활성화된 인덱스 (열)")) -> (element=w1529:string[])  [unwired: 1 in]
        n499 = Multiply(x=w1541, y=10) -> (x*y=w1539:i32)
        n500 = Not Equal?(x=w1511, y="0") -> (x != y?=w1506:bool)
        n501 = Number To Decimal String(number=w1539) -> (decimal integer string=w1538:string)  [unwired: 1 in]
        n502 = Search 1D Array(1D array=w1529, element=w1524) -> (index of element=w1528:i32)  [unwired: 1 in]
        n503 = Index Array(array=w1526, index (row)=w1528, index (col)=1 ("비활성화된 인덱스 (열)")) -> (element=w1525:string)
        n504 = Select(t=w1511, s=w1506, f="0.1" ("t")) -> (s? t:f=w1513:string)
        n505 = Select(t=w1509, s=w1506, f="N·m" ("t")) -> (s? t:f=w1508:string)
        n506 = Build Array(w1516, w1517, w1505, w1505, w1505, w1505, w1513, w1508) -> (w1515:string[])
        n507 = Build Array(w1538, w1536, w1516, w1534, w1533, w1532, w1524, w1524, w1531, w1525, w1510, w1510, w1510, w1510, w1510, w1510, w1510, w1510, w1523, w1522, w1521, w1520, w1519) -> (w1535:string[])
      }
    }
    frame "20303-0" {
      w1543 = 0 ("비활성화된 인덱스 (열)")
      n508 = Index Array(array=w1550, index (col)=w1543) -> (element=w1551:string[])  [unwired: 1 in]
      n509 = Increment(x=w1543) -> (x+1=w1542:i32)
      n510 = call-poly "Array Deduplication.vi"("배열 in"=w1551) -> ("배열 out"=w1549:string[])  [unwired: 9 in, 1 out]
      n511 = for {
        tunnel: w1550 -> [w1569]
        tunnel: w1549 -> [w1568] mode=indexing
        tunnel: [w1558] -> w1548 mode=indexing
        tunnel: w1543 -> [w1557]
        tunnel: w1542 -> [w1556]
        n512 = call "Data Class_2D Str.vi"("인덱스"=w1557, "DATA 입력"=w1569, "검색 문자열"=w1568) -> ("DATA 출력"=w1565:string[][])  [unwired: 4 in, 4 out]
        n513 = Index Array(array=w1565, index (col)=w1556) -> (element=w1567:string[])  [unwired: 1 in]
        n514 = Fract/Exp String To Number(string=w1567) -> (number=w1566:dbl[])  [unwired: 3 in, 1 out]
        n515 = Array Max & Min(array=w1566) -> (max index (indices)=w1564:i32)  [unwired: 3 out]
        n516 = Index Array(array=w1565, index (row) #1=w1564, index (col) #1=w1557) -> (element #1=w1560:string, element #2=w1562:string, element #3=w1561:string)  [unwired: 4 in]
        n517 = Format Into String(format string="%s %s" ("포맷 문자열"), w1562, w1561) -> (resulting string=w1559:string)  [unwired: 2 in, 1 out]
        n518 = Build Array(w1560, w1559) -> (w1558:string[])
      }
      n519 = Unbundle By Name(w1555) -> ("추가문자열"=w1554:string, "형식"=w1553:string, "옵션"=w1552:string)
      n520 = for {
        tunnel: w1550 -> [w1582] mode=indexing
        tunnel: w1546 -> [w1580]
        tunnel: w1554 -> [w1599]
        tunnel: w1553 -> [w1598]
        tunnel: w1552 -> [w1597]
        tunnel: [w1579] -> w1545 mode=indexing
        tunnel: w1548 -> [w1590]
        tunnel: [w1600] -> w1547 mode=indexing
        i -> [w1606]
        w1574 = "" ("원소")
        w1593 = ""  # C4~C10
        w1596 = "0"  # 엑셀문서명(C1)
        n521 = Index Array(array=w1582) -> (element #1=w1588:string, element #2=w1587:string, element #3=w1586:string, element #4=w1585:string, element #5=w1584:string, element #6=w1583:string)  [unwired: 6 in]
        n522 = Index Array(array=w1582) -> (element #1=w1581:string, element #2=w1575:string, element #3=w1573:string)  [unwired: 3 in]
        n523 = String Subset(string=w1580, length (rest)=5 ("길이(나머지)")) -> (substring=w1601:string)  [unwired: 1 in]
        n524 = Index Array(array=w1590, index (col)=0 ("비활성화된 인덱스 (열)")) -> (element=w1594:string[])  [unwired: 1 in]
        n525 = Multiply(x=w1606, y=10) -> (x*y=w1604:i32)
        n526 = Not Equal?(x=w1575, y="0") -> (x != y?=w1571:bool)
        n527 = Number To Decimal String(number=w1604) -> (decimal integer string=w1603:string)  [unwired: 1 in]
        n528 = Search 1D Array(1D array=w1594, element=w1588) -> (index of element=w1592:i32)  [unwired: 1 in]
        n529 = Index Array(array=w1590, index (row)=w1592, index (col)=1 ("비활성화된 인덱스 (열)")) -> (element=w1589:string)
        n530 = Select(t=w1575, s=w1571, f="0.05" ("t")) -> (s? t:f=w1577:string)
        n531 = Select(t=w1573, s=w1571, f="N·m") -> (s? t:f=w1572:string)
        n532 = Build Array(w1580, w1581, w1574, w1574, w1574, w1574, w1577, w1572) -> (w1579:string[])
        n533 = Build Array(w1603, w1601, w1580, w1599, w1598, w1597, w1588, w1588, w1596, w1589, w1585, w1593, w1593, w1593, w1593, w1593, w1593, w1593, w1587, w1586, w1585, w1584, w1583) -> (w1600:string[])
      }
    }
    frame "20406-0" {
      w1608 = 1 ("비활성화된 인덱스 (열)")
      n534 = Index Array(array=w1615, index (col)=w1608) -> (element=w1616:string[])  [unwired: 1 in]
      n535 = Increment(x=w1608) -> (x+1=w1607:i32)
      n536 = call-poly "Array Deduplication.vi"("배열 in"=w1616) -> ("배열 out"=w1614:string[])  [unwired: 9 in, 1 out]
      n537 = for {
        tunnel: w1615 -> [w1640]
        tunnel: w1614 -> [w1639] mode=indexing
        tunnel: [w1632] -> w1613 mode=indexing
        tunnel: w1608 -> [w1630]
        tunnel: w1607 -> [w1621]
        w1629 = "%s %s" ("포맷 문자열")
        n538 = call "Data Class_2D Str.vi"("인덱스"=w1630, "DATA 입력"=w1640, "검색 문자열"=w1639) -> ("DATA 출력"=w1638:string[][])  [unwired: 4 in, 4 out]
        n539 = Index Array(array=w1638, index (col) #1=w1621) -> (element #1=w1625:string[], element #2=w1624:string[])  [unwired: 3 in]
        n540 = for {
          tunnel: w1625 -> [w1644] mode=indexing
          tunnel: w1624 -> [w1643] mode=indexing
          tunnel: "kPa abs." -> [w1642]
          tunnel: [w1641] -> w1622 mode=indexing
          n541 = call "Unit Conversion.vi"("환산단위"=w1642, "입력단위"=w1643, "입력값"=w1644) -> ("환산값 (DBL)"=w1641:dbl)  [unwired: 3 in, 5 out]
        }
        n542 = Array Max & Min(array=w1622) -> (max index (indices)=w1637:i32, min index (indices)=w1631:i32)  [unwired: 2 out]
        n543 = Index Array(array=w1638, index (row) #1=w1637, index (col) #1=w1630, index (row) #4=w1631, index (col) #4=w1630) -> (element #1=w1634:string, element #2=w1636:string, element #3=w1635:string, element #5=w1627:string, element #6=w1626:string)  [unwired: 8 in, 1 out]
        n544 = Format Into String(format string=w1629, w1636, w1635) -> (resulting string=w1633:string)  [unwired: 2 in, 1 out]
        n545 = Format Into String(format string=w1629, w1627, w1626) -> (resulting string=w1628:string)  [unwired: 2 in, 1 out]
        n546 = Build Array(w1634, w1633, w1628) -> (w1632:string[])
      }
      n547 = Unbundle By Name(w1620) -> ("추가문자열"=w1619:string, "형식"=w1618:string, "옵션"=w1617:string)
      n548 = for {
        tunnel: w1615 -> [w1653] mode=indexing
        tunnel: w1611 -> [w1654]
        tunnel: w1619 -> [w1671]
        tunnel: w1618 -> [w1670]
        tunnel: w1617 -> [w1669]
        tunnel: [w1652] -> w1610 mode=indexing
        tunnel: w1613 -> [w1661]
        tunnel: [w1672] -> w1612 mode=indexing
        i -> [w1678]
        w1645 = "" ("원소")
        w1663 = ""  # C3~C10
        w1667 = "0"  # 엑셀문서명(C1)
        n549 = Index Array(array=w1653) -> (element #1=w1668:string, element #2=w1664:string, element #3=w1659:string, element #4=w1658:string, element #5=w1657:string, element #6=w1656:string, element #7=w1655:string)  [unwired: 7 in]
        n550 = Index Array(array=w1653) -> (element #1=w1651:string, element #3=w1650:string, element #4=w1649:string)  [unwired: 4 in, 1 out]
        n551 = String Subset(string=w1654, length (rest)=5 ("길이(나머지)")) -> (substring=w1673:string)  [unwired: 1 in]
        n552 = Index Array(array=w1661, index (col)=0 ("비활성화된 인덱스 (열)")) -> (element=w1665:string[])  [unwired: 1 in]
        n553 = Multiply(x=w1678, y=10) -> (x*y=w1676:i32)
        n554 = Number To Decimal String(number=w1676) -> (decimal integer string=w1675:string)  [unwired: 1 in]
        n555 = Search 1D Array(1D array=w1665, element=w1664) -> (index of element=w1648:i32)  [unwired: 1 in]
        n556 = Index Array(array=w1661, index (row) #1=w1648, index (col) #1=1 ("비활성화된 인덱스 (열)"), index (row) #2=w1648, index (col) #2=2 ("비활성화된 인덱스 (열)")) -> (element #1=w1660:string, element #2=w1646:string)
        n557 = Build Array(w1654, w1651, w1645, w1645, w1645, w1645, w1650, w1649) -> (w1652:string[])
        n558 = Build Array(w1675, w1673, w1654, w1671, w1670, w1669, w1668, w1664, w1667, w1660, w1646, w1663, w1663, w1663, w1663, w1663, w1663, w1663, w1659, w1658, w1657, w1656, w1655) -> (w1672:string[])
      }
    }
    frame "20408-0" {
      w1680 = 1 ("비활성화된 인덱스 (열)")
      n559 = Index Array(array=w1687, index (col)=w1680) -> (element=w1688:string[])  [unwired: 1 in]
      n560 = Increment(x=w1680) -> (x+1=w1679:i32)
      n561 = call-poly "Array Deduplication.vi"("배열 in"=w1688) -> ("배열 out"=w1686:string[])  [unwired: 9 in, 1 out]
      n562 = for {
        tunnel: w1687 -> [w1712]
        tunnel: w1686 -> [w1711] mode=indexing
        tunnel: [w1704] -> w1685 mode=indexing
        tunnel: w1680 -> [w1702]
        tunnel: w1679 -> [w1693]
        w1701 = "%s %s" ("포맷 문자열")
        n563 = call "Data Class_2D Str.vi"("인덱스"=w1702, "DATA 입력"=w1712, "검색 문자열"=w1711) -> ("DATA 출력"=w1710:string[][])  [unwired: 4 in, 4 out]
        n564 = Index Array(array=w1710, index (col) #1=w1693) -> (element #1=w1697:string[], element #2=w1696:string[])  [unwired: 3 in]
        n565 = for {
          tunnel: w1697 -> [w1716] mode=indexing
          tunnel: w1696 -> [w1715] mode=indexing
          tunnel: "kPa" -> [w1714]
          tunnel: [w1713] -> w1694 mode=indexing
          n566 = call "Unit Conversion.vi"("환산단위"=w1714, "입력단위"=w1715, "입력값"=w1716) -> ("환산값 (DBL)"=w1713:dbl)  [unwired: 3 in, 5 out]
        }
        n567 = Array Max & Min(array=w1694) -> (max index (indices)=w1709:i32, min index (indices)=w1703:i32)  [unwired: 2 out]
        n568 = Index Array(array=w1710, index (row) #1=w1709, index (col) #1=w1702, index (row) #4=w1703, index (col) #4=w1702) -> (element #1=w1706:string, element #2=w1708:string, element #3=w1707:string, element #5=w1699:string, element #6=w1698:string)  [unwired: 8 in, 1 out]
        n569 = Format Into String(format string=w1701, w1708, w1707) -> (resulting string=w1705:string)  [unwired: 2 in, 1 out]
        n570 = Format Into String(format string=w1701, w1699, w1698) -> (resulting string=w1700:string)  [unwired: 2 in, 1 out]
        n571 = Build Array(w1706, w1705, w1700) -> (w1704:string[])
      }
      n572 = Unbundle By Name(w1692) -> ("추가문자열"=w1691:string, "형식"=w1690:string, "옵션"=w1689:string)
      n573 = for {
        tunnel: w1687 -> [w1725] mode=indexing
        tunnel: w1683 -> [w1726]
        tunnel: w1691 -> [w1743]
        tunnel: w1690 -> [w1742]
        tunnel: w1689 -> [w1741]
        tunnel: [w1724] -> w1682 mode=indexing
        tunnel: w1685 -> [w1733]
        tunnel: [w1744] -> w1684 mode=indexing
        i -> [w1750]
        w1717 = "" ("원소")
        w1735 = ""  # C3~C10
        w1739 = "0"  # 엑셀문서명(C1)
        n574 = Index Array(array=w1725) -> (element #1=w1740:string, element #2=w1736:string, element #3=w1731:string, element #4=w1730:string, element #5=w1729:string, element #6=w1728:string, element #7=w1727:string)  [unwired: 7 in]
        n575 = Index Array(array=w1725) -> (element #1=w1723:string, element #3=w1722:string, element #4=w1721:string)  [unwired: 4 in, 1 out]
        n576 = String Subset(string=w1726, length (rest)=5 ("길이(나머지)")) -> (substring=w1745:string)  [unwired: 1 in]
        n577 = Index Array(array=w1733, index (col)=0 ("비활성화된 인덱스 (열)")) -> (element=w1737:string[])  [unwired: 1 in]
        n578 = Multiply(x=w1750, y=10) -> (x*y=w1748:i32)
        n579 = Number To Decimal String(number=w1748) -> (decimal integer string=w1747:string)  [unwired: 1 in]
        n580 = Search 1D Array(1D array=w1737, element=w1736) -> (index of element=w1720:i32)  [unwired: 1 in]
        n581 = Index Array(array=w1733, index (row) #1=w1720, index (col) #1=1 ("비활성화된 인덱스 (열)"), index (row) #2=w1720, index (col) #2=2 ("비활성화된 인덱스 (열)")) -> (element #1=w1732:string, element #2=w1718:string)
        n582 = Build Array(w1726, w1723, w1717, w1717, w1717, w1717, w1722, w1721) -> (w1724:string[])
        n583 = Build Array(w1747, w1745, w1726, w1743, w1742, w1741, w1740, w1736, w1739, w1732, w1718, w1735, w1735, w1735, w1735, w1735, w1735, w1735, w1731, w1730, w1729, w1728, w1727) -> (w1744:string[])
      }
    }
    frame "20409-0" {
      w1752 = 1 ("비활성화된 인덱스 (열)")
      n584 = Index Array(array=w1759, index (col)=w1752) -> (element=w1760:string[])  [unwired: 1 in]
      n585 = Increment(x=w1752) -> (x+1=w1751:i32)
      n586 = call-poly "Array Deduplication.vi"("배열 in"=w1760) -> ("배열 out"=w1758:string[])  [unwired: 9 in, 1 out]
      n587 = for {
        tunnel: w1759 -> [w1782]
        tunnel: w1758 -> [w1781] mode=indexing
        tunnel: [w1773] -> w1757 mode=indexing
        tunnel: w1752 -> [w1771]
        tunnel: w1751 -> [w1765]
        w1767 = "%s %s" ("포맷 문자열")
        n588 = call "Data Class_2D Str.vi"("인덱스"=w1771, "DATA 입력"=w1782, "검색 문자열"=w1781) -> ("DATA 출력"=w1779:string[][])  [unwired: 4 in, 4 out]
        n589 = Index Array(array=w1779, index (col)=w1765) -> (element=w1780:string[])  [unwired: 1 in]
        n590 = Fract/Exp String To Number(string=w1780) -> (number=w1772:dbl[])  [unwired: 3 in, 1 out]
        n591 = Array Max & Min(array=w1772) -> (max index (indices)=w1778:i32, min index (indices)=w1770:i32)  [unwired: 2 out]
        n592 = Index Array(array=w1779, index (row) #1=w1778, index (col) #1=w1771, index (row) #4=w1770, index (col) #4=w1771) -> (element #1=w1775:string, element #2=w1777:string, element #3=w1776:string, element #5=w1769:string, element #6=w1768:string)  [unwired: 8 in, 1 out]
        n593 = Format Into String(format string=w1767, w1777, w1776) -> (resulting string=w1774:string)  [unwired: 2 in, 1 out]
        n594 = Format Into String(format string=w1767, w1769, w1768) -> (resulting string=w1766:string)  [unwired: 2 in, 1 out]
        n595 = Build Array(w1775, w1774, w1766) -> (w1773:string[])
      }
      n596 = Unbundle By Name(w1764) -> ("추가문자열"=w1763:string, "형식"=w1762:string, "옵션"=w1761:string)
      n597 = for {
        tunnel: w1759 -> [w1794] mode=indexing
        tunnel: w1755 -> [w1795]
        tunnel: w1763 -> [w1810]
        tunnel: w1762 -> [w1809]
        tunnel: w1761 -> [w1808]
        tunnel: [w1793] -> w1754 mode=indexing
        tunnel: w1757 -> [w1800]
        tunnel: [w1811] -> w1756 mode=indexing
        i -> [w1817]
        w1783 = "" ("원소")
        w1802 = ""  # C6~C10
        w1806 = "0"  # 엑셀문서명(C1)
        n598 = Index Array(array=w1794) -> (element #1=w1807:string, element #2=w1803:string, element #3=w1787:string, element #4=w1788:string, element #5=w1798:string, element #6=w1797:string, element #7=w1796:string)  [unwired: 7 in]
        n599 = Index Array(array=w1794) -> (element #1=w1792:string, element #4=w1791:string)  [unwired: 4 in, 2 out]
        n600 = String Subset(string=w1795, length (rest)=5 ("길이(나머지)")) -> (substring=w1812:string)  [unwired: 1 in]
        n601 = Index Array(array=w1800, index (col)=0 ("비활성화된 인덱스 (열)")) -> (element=w1804:string[])  [unwired: 1 in]
        n602 = Multiply(x=w1817, y=10) -> (x*y=w1815:i32)
        n603 = Number To Decimal String(number=w1815) -> (decimal integer string=w1814:string)  [unwired: 1 in]
        n604 = Search 1D Array(1D array=w1804, element=w1803) -> (index of element=w1786:i32)  [unwired: 1 in]
        n605 = Search and Replace String(input string=w1787, search string="-" ("검색 문자열")) -> (result string=w1789:string)  [unwired: 6 in, 3 out]
        n606 = Index Array(array=w1800, index (row) #1=w1786, index (col) #1=1 ("비활성화된 인덱스 (열)"), index (row) #2=w1786, index (col) #2=2 ("비활성화된 인덱스 (열)")) -> (element #1=w1799:string, element #2=w1784:string)
        n607 = Build Array(w1795, w1792, w1783, w1783, w1783, w1783, w1789, w1791) -> (w1793:string[])
        n608 = Build Array(w1814, w1812, w1795, w1810, w1809, w1808, w1807, w1803, w1806, w1799, w1784, w1787, w1788, w1802, w1802, w1802, w1802, w1802, w1789, w1788, w1798, w1797, w1796) -> (w1811:string[])
      }
    }
    frame "20413-0" {
      w1819 = 1 ("비활성화된 인덱스 (열)")
      n609 = Index Array(array=w1826, index (col)=w1819) -> (element=w1827:string[])  [unwired: 1 in]
      n610 = Increment(x=w1819) -> (x+1=w1818:i32)
      n611 = call-poly "Array Deduplication.vi"("배열 in"=w1827) -> ("배열 out"=w1825:string[])  [unwired: 9 in, 1 out]
      n612 = for {
        tunnel: w1826 -> [w1845]
        tunnel: w1825 -> [w1844] mode=indexing
        tunnel: [w1835] -> w1824 mode=indexing
        tunnel: w1819 -> [w1834]
        tunnel: w1818 -> [w1832]
        n613 = call "Data Class_2D Str.vi"("인덱스"=w1834, "DATA 입력"=w1845, "검색 문자열"=w1844) -> ("DATA 출력"=w1841:string[][])  [unwired: 4 in, 4 out]
        n614 = Index Array(array=w1841, index (col)=w1832) -> (element=w1843:string[])  [unwired: 1 in]
        n615 = Fract/Exp String To Number(string=w1843) -> (number=w1842:dbl[])  [unwired: 3 in, 1 out]
        n616 = Array Max & Min(array=w1842) -> (min index (indices)=w1833:i32)  [unwired: 3 out]
        n617 = Index Array(array=w1841, index (row) #1=w1833, index (col) #1=w1834) -> (element #1=w1837:string, element #2=w1839:string, element #3=w1838:string)  [unwired: 4 in]
        n618 = Format Into String(format string="%s %s" ("포맷 문자열"), w1839, w1838) -> (resulting string=w1836:string)  [unwired: 2 in, 1 out]
        n619 = Build Array(w1837, w1836) -> (w1835:string[])
      }
      n620 = Unbundle By Name(w1831) -> ("추가문자열"=w1830:string, "형식"=w1829:string, "옵션"=w1828:string)
      n621 = for {
        tunnel: w1826 -> [w1851] mode=indexing
        tunnel: w1822 -> [w1852]
        tunnel: w1830 -> [w1870]
        tunnel: w1829 -> [w1869]
        tunnel: w1828 -> [w1868]
        tunnel: [w1850] -> w1821 mode=indexing
        tunnel: w1824 -> [w1859]
        tunnel: [w1871] -> w1823 mode=indexing
        i -> [w1877]
        w1846 = "" ("원소")
        w1862 = ""  # C3~C10
        w1866 = "0"  # 엑셀문서명(C1)
        n622 = Index Array(array=w1851) -> (element #1=w1867:string, element #2=w1863:string, element #3=w1857:string, element #4=w1856:string, element #5=w1855:string, element #6=w1854:string, element #7=w1853:string)  [unwired: 7 in]
        n623 = Index Array(array=w1851) -> (element #1=w1849:string, element #3=w1848:string, element #4=w1847:string)  [unwired: 4 in, 1 out]
        n624 = String Subset(string=w1852, length (rest)=5 ("길이(나머지)")) -> (substring=w1872:string)  [unwired: 1 in]
        n625 = Index Array(array=w1859, index (col)=0 ("비활성화된 인덱스 (열)")) -> (element=w1864:string[])  [unwired: 1 in]
        n626 = Multiply(x=w1877, y=10) -> (x*y=w1875:i32)
        n627 = Search 1D Array(1D array=w1864, element=w1863) -> (index of element=w1861:i32)  [unwired: 1 in]
        n628 = Number To Decimal String(number=w1875) -> (decimal integer string=w1874:string)  [unwired: 1 in]
        n629 = Index Array(array=w1859, index (row)=w1861, index (col)=1 ("비활성화된 인덱스 (열)")) -> (element=w1858:string)
        n630 = Build Array(w1852, w1849, w1846, w1846, w1846, w1846, w1848, w1847) -> (w1850:string[])
        n631 = Build Array(w1874, w1872, w1852, w1870, w1869, w1868, w1867, w1863, w1866, w1858, w1862, w1862, w1862, w1862, w1862, w1862, w1862, w1862, w1857, w1856, w1855, w1854, w1853) -> (w1871:string[])
      }
    }
    frame "20414-0" {
      w1879 = 1 ("비활성화된 인덱스 (열)")
      n632 = Index Array(array=w1886, index (col)=w1879) -> (element=w1887:string[])  [unwired: 1 in]
      n633 = Increment(x=w1879) -> (x+1=w1878:i32)
      n634 = call-poly "Array Deduplication.vi"("배열 in"=w1887) -> ("배열 out"=w1885:string[])  [unwired: 9 in, 1 out]
      n635 = for {
        tunnel: w1886 -> [w1905]
        tunnel: w1885 -> [w1904] mode=indexing
        tunnel: [w1895] -> w1884 mode=indexing
        tunnel: w1879 -> [w1894]
        tunnel: w1878 -> [w1892]
        n636 = call "Data Class_2D Str.vi"("인덱스"=w1894, "DATA 입력"=w1905, "검색 문자열"=w1904) -> ("DATA 출력"=w1901:string[][])  [unwired: 4 in, 4 out]
        n637 = Index Array(array=w1901, index (col)=w1892) -> (element=w1903:string[])  [unwired: 1 in]
        n638 = Fract/Exp String To Number(string=w1903) -> (number=w1902:dbl[])  [unwired: 3 in, 1 out]
        n639 = Array Max & Min(array=w1902) -> (max index (indices)=w1893:i32)  [unwired: 3 out]
        n640 = Index Array(array=w1901, index (row) #1=w1893, index (col) #1=w1894) -> (element #1=w1897:string, element #2=w1899:string, element #3=w1898:string)  [unwired: 4 in]
        n641 = Format Into String(format string="%s %s" ("포맷 문자열"), w1899, w1898) -> (resulting string=w1896:string)  [unwired: 2 in, 1 out]
        n642 = Build Array(w1897, w1896) -> (w1895:string[])
      }
      n643 = Unbundle By Name(w1891) -> ("추가문자열"=w1890:string, "형식"=w1889:string, "옵션"=w1888:string)
      n644 = for {
        tunnel: w1886 -> [w1918] mode=indexing
        tunnel: w1882 -> [w1919]
        tunnel: w1890 -> [w1932]
        tunnel: w1889 -> [w1931]
        tunnel: w1888 -> [w1930]
        tunnel: [w1917] -> w1881 mode=indexing
        tunnel: w1884 -> [w1921]
        tunnel: [w1933] -> w1883 mode=indexing
        i -> [w1939]
        w1906 = "" ("원소")
        w1924 = ""  # C5~C10
        w1928 = "0"  # 엑셀문서명(C1)
        n645 = Index Array(array=w1918) -> (element #1=w1929:string, element #2=w1925:string, element #3=w1913:string, element #4=w1912:string, element #5=w1911:string, element #6=w1910:string, element #7=w1909:string, element #8=w1908:string, element #9=w1907:string)  [unwired: 9 in]
        n646 = Index Array(array=w1918) -> (element #1=w1916:string, element #3=w1915:string, element #4=w1914:string)  [unwired: 4 in, 1 out]
        n647 = String Subset(string=w1919, length (rest)=5 ("길이(나머지)")) -> (substring=w1934:string)  [unwired: 1 in]
        n648 = Index Array(array=w1921, index (col)=0 ("비활성화된 인덱스 (열)")) -> (element=w1926:string[])  [unwired: 1 in]
        n649 = Multiply(x=w1939, y=10) -> (x*y=w1937:i32)
        n650 = Search 1D Array(1D array=w1926, element=w1925) -> (index of element=w1923:i32)  [unwired: 1 in]
        n651 = Number To Decimal String(number=w1937) -> (decimal integer string=w1936:string)  [unwired: 1 in]
        n652 = Index Array(array=w1921, index (row)=w1923, index (col)=1 ("비활성화된 인덱스 (열)")) -> (element=w1920:string)
        n653 = Build Array(w1919, w1916, w1906, w1906, w1906, w1906, w1915, w1914) -> (w1917:string[])
        n654 = Build Array(w1936, w1934, w1919, w1932, w1931, w1930, w1929, w1925, w1928, w1920, w1913, w1912, w1924, w1924, w1924, w1924, w1924, w1924, w1911, w1910, w1909, w1908, w1907) -> (w1933:string[])
      }
    }
    frame "40419-0" {
      # "9, 없음"
      n655 = Unbundle By Name(w1948) -> ("추가문자열"=w1947:string, "형식"=w1946:string, "옵션"=w1945:string)
      n656 = for {
        tunnel: w1944 -> [w1959] mode=indexing
        tunnel: w1942 -> [w1960]
        tunnel: w1947 -> [w1971]
        tunnel: w1946 -> [w1970]
        tunnel: w1945 -> [w1969]
        tunnel: [w1958] -> w1941 mode=indexing
        tunnel: [w1974] -> w1943 mode=indexing
        i -> [w1978]
        w1954 = ""
        w1963 = ""  # C3~C10
        w1967 = "0"  # 엑셀문서명(C1)
        n657 = Index Array(array=w1959) -> (element #1=w1968:string, element #2=w1966:string, element #3=w1965:string, element #4=w1964:string, element #5=w1962:string, element #6=w1961:string, element #7=w1957:string, element #8=w1956:string, element #9=w1955:string)  [unwired: 9 in]
        n658 = Index Array(array=w1959) -> (element #1=w1949:string, element #3=w1953:string, element #4=w1952:string, element #5=w1951:string, element #6=w1950:string)  [unwired: 6 in, 1 out]
        n659 = String Subset(string=w1960, length (rest)=5 ("길이(나머지)")) -> (substring=w1973:string)  [unwired: 1 in]
        n660 = Multiply(x=w1978, y=10) -> (x*y=w1976:i32)
        n661 = Number To Decimal String(number=w1976) -> (decimal integer string=w1972:string)  [unwired: 1 in]
        n662 = Build Array(w1960, w1949, w1954, w1954, w1953, w1952, w1951, w1950) -> (w1958:string[])
        n663 = Build Array(w1972, w1973, w1960, w1971, w1970, w1969, w1968, w1963, w1967, w1966, w1965, w1964, w1963, w1963, w1963, w1963, w1963, w1963, w1962, w1961, w1957, w1956, w1955) -> (w1974:string[])
      }
    }
    frame Default {
      n664 = xnode "에러 링"("파라미터 0"=w1979) -> ("에러 출력"=w1981:errorcluster)
    }
  }
  "배열출력" <- w30
  n665 = call "sub_CMC Match.vi"("error in (no error)"=w20, "DATA IN"=w16, "CMC IN"="CMC") -> ("error out"=w19:errorcluster, "에러?"=→"에러?":bool, "CMC Out"=w18:string[][])  [unwired: 6 in]
  n666 = for {
    tunnel: w5 -> [w1996] mode=indexing
    tunnel: w18 -> [w1995] mode=indexing
    tunnel: [w1989] -> w21 mode=indexing
    n667 = Index Array(array=w1995, index #1=18 ("인덱스")) -> (element #1=w1993:string, element #3=w1992:string)  [unwired: 2 in, 1 out]
    n668 = Format Into String(format string="%s %s" ("포맷 문자열"), w1993, w1992) -> (resulting string=w1991:string)  [unwired: 2 in, 1 out]
    n669 = Insert Into Array(array=w1996, new element=w1991) -> (w1989:string[])  [unwired: 1 in]
  }
  n670 = call-poly "Cell Spacing.vi"("error in"=w19, "Data in"=w21, "테이블 참조 in"=w24) -> ("error out"=→"에러 출력":errorcluster)  [unwired: 6 in, 2 out]
